vi "FieldMillTOBoltek.vi"() -> ()   [LabVIEW 2010]
uses:
  <vilib>/Utility/error.llb/DialogType.ctl
  <vilib>/Platform/TimedLoop/XDataNode/XDataNode.xnode
  <vilib>/Platform/TimedLoop/XDataNode/timing_clust.ctl
  <vilib>/Platform/TimedLoop/XDataNode/nitl_modes.ctl
  <vilib>/Platform/TimedLoop/XDataNode/wakeup.ctl
  <vilib>/Instr/_visa.llb/VISA Configure Serial Port (Instr).vi
  <vilib>/Utility/file.llb/Write To Spreadsheet File (DBL).vi
  <vilib>/Utility/file.llb/Read From Spreadsheet File (DBL).vi
  <vilib>/Platform/TimedLoop/XDataNode/XDNodeRunTimeDep.lvlib
panel:
  out "6":bool
  out "12":bool
  out "24":bool
  out "37":bool
  out "6_R":dbl(knob) caption="6" scale=0.0..10.0
  out "12_R":dbl(knob) caption="12" scale=0.0..10.0
  out "24_R":dbl(knob) caption="24" scale=0.0..10.0
  out "37_R":dbl(knob) caption="37" scale=0.0..10.0
  out "Strike distance Km":dbl
  in  "6 2":bool
  in  "12 2":bool
  in  "24 2":bool
  in  "37 2":bool
  out "kV/m tampone":dbl
  out "BOL IN":bool
  out "Offset":dbl format="%.1f"
  out "BOL OUT":bool
  out "SOCKET":bool
  out "FTP":bool
  out "Inver. sign":bool=TRUE
  out "Mediated v..":bool
  in  "FEM_ON_OFF":string
  out "Offset_p":i32 format="%.1f"
  out "Inverted_p":string
  out "Mediated_p":string
  out "User:":string
  out "Min":sgl caption="Min hour" format="%.3f"
  out "Max":sgl caption="Max hour" format="%.3f"
  out "Min":sgl caption="Min 10Min" format="%.3f"
  out "Max":sgl caption="Max 10Min" format="%.3f"
  out "Min":sgl caption="Min Midnight" format="%.3f"
  out "Max":sgl caption="Max Midnight" format="%.3f"
  out "Station Info graph":string
  out "Time & Date 2":timestamp format="%<%x>T"
  out "Time & Date":timestamp format="%<%H:%M:%S>T"
  out "String Alarm":string
  in  "About":bool
  in  "temp.csv midnight":bool
  out "remoteinfopath":string
  in  "Graph":bool=TRUE
  out "CLOSE COMMBOL":errorcluster
  out "CLOSE COMMFEM":errorcluster
  in  "COMMBOL ON_OFF":string
  out "Array via socket":string[](array[string])
  out "Multi socket String":string
  out "Alarm VHf counter":i32
  in  "Numero ripetizioni alarm VHf":i32
  out "In ripetizione VHf ?":bool
  out "Alarm Hf counter":i32
  in  "Numero ripetizioni alarm Hf":i32
  out "FEM Graph_IMAGES":cluster{dbl, dbl}[](graph) caption="FEM software - 5 min Graph - 15-05-13 / 11:59:33 ---- [ ROMA(Italy) - 41.995461 - 12.546161 - http://www.kwos.org ]"
  in  "SOCKET ON_OFF":string
  in  "Socket Port":u16=6340 min=1025 step=1
  out "Socket String":string
  out "24hour graph string":string
  out "4hour graph string":string
  out "1hour graph string":string
  out "LiveGraph string":string
  in  "Path24hourFile":path
  in  "Path4hourFile":path
  in  "Path1hourFile":path
  in  "PathCurrentFile":path
  in  "Ripetizioni alarm VHf":bool
  out "In allarme VHf ?":bool
  out "In allarme Hf ?":bool
  in  "Ripetizioni alarm Hf":bool
  out "Seconds Very High field alarm":sgl=1.0 format="%#_1f"
  out "Very High field alarm":sgl=5.0 format="%#_1f"
  out "Seconds High field alarm":sgl=1.0 format="%#_1f"
  out "High field alarm":sgl=1.0 format="%#_1f"
  in  "MENU ALARMS":bool
  out "Offset":dbl
  in  "Time Knob":u32(knob)=320 scale=300.0..86400.0 scale format="%#.0g"
  out "kV/m":string caption="kV/m display"
  out "FEM Graph":cluster{dbl, dbl}[](graph) caption="FEM software - 24 hours Graph - 23-10-09 / 18:44:02"
  in  "kV/m knob":sgl(knob)=1.0 scale=0.5..20.0
  out "data string 3":string
  out "data string FEM":string
  out "Mediated v.":bool
  out "Inversion sign":bool=TRUE caption="Inversion sign 2"
  out "FTP":bool
  in  "MENU INTERNET":bool
  in  "MENU FILTERS":bool
  out "Errori lettura file di configurazione":errorcluster={"status"=FALSE, "code"=0, "source"="Read File+ (string): Read File"}
  out "4 valori per media in array":dbl[](array[numeric]) format="%0.2f"
  in  "remotepath":string
  in  "passftp":string
  in  "loginftp":string
  in  "ftpsite":string
  in  "seconds":u32=30 min=30 max=3600 step=30
  in  "port number 2":refnum<visa-resource-name>="COM16"
  in  "parity 2":enum16{"None", "Odd", "Even", "Mark", "Space"}(ring)
  in  "port number":refnum<visa-resource-name>="COM5"
  in  "parity":enum16{"None", "Odd", "Even", "Mark", "Space"}(ring)
  out "COM err msg: 2":string="No Error"
  out "Boolean 2":bool
  in  "data bit 2":i32=8
  in  "baud rate 2":u32=9600
  out "kV/m":string
  out "mV":string
  in  "data bit":i32=8
  out "Boolean":bool
  in  "baud rate":u32=9600
  out "COM err msg:":string="No Error"
  # "E-Field Mill"
  # "kV/m"
  # "mV"
  # "=>"
  # "Sezione TEST"
  # "E-Field Mill Software"
  # "COMMFEM"
  # "COMMBOL"
  # "FILTRI"
  # "No"
  # "Yes"
  # "Inv"
  # "Norm"
  # "INTERNET"
  # "FTP TRANSFER ON/OFF"
  # "ALLARMI"
  # "Strike distance evaluation"
  # "Km"
  # "Last 10 min"
  # "Last hour"
  # "From midnight"
  # "ALERT Indicator"
  # "FEEDBACK RS232 => BOLTEK"
  # "FEEDBACK RS232 <= FEM"
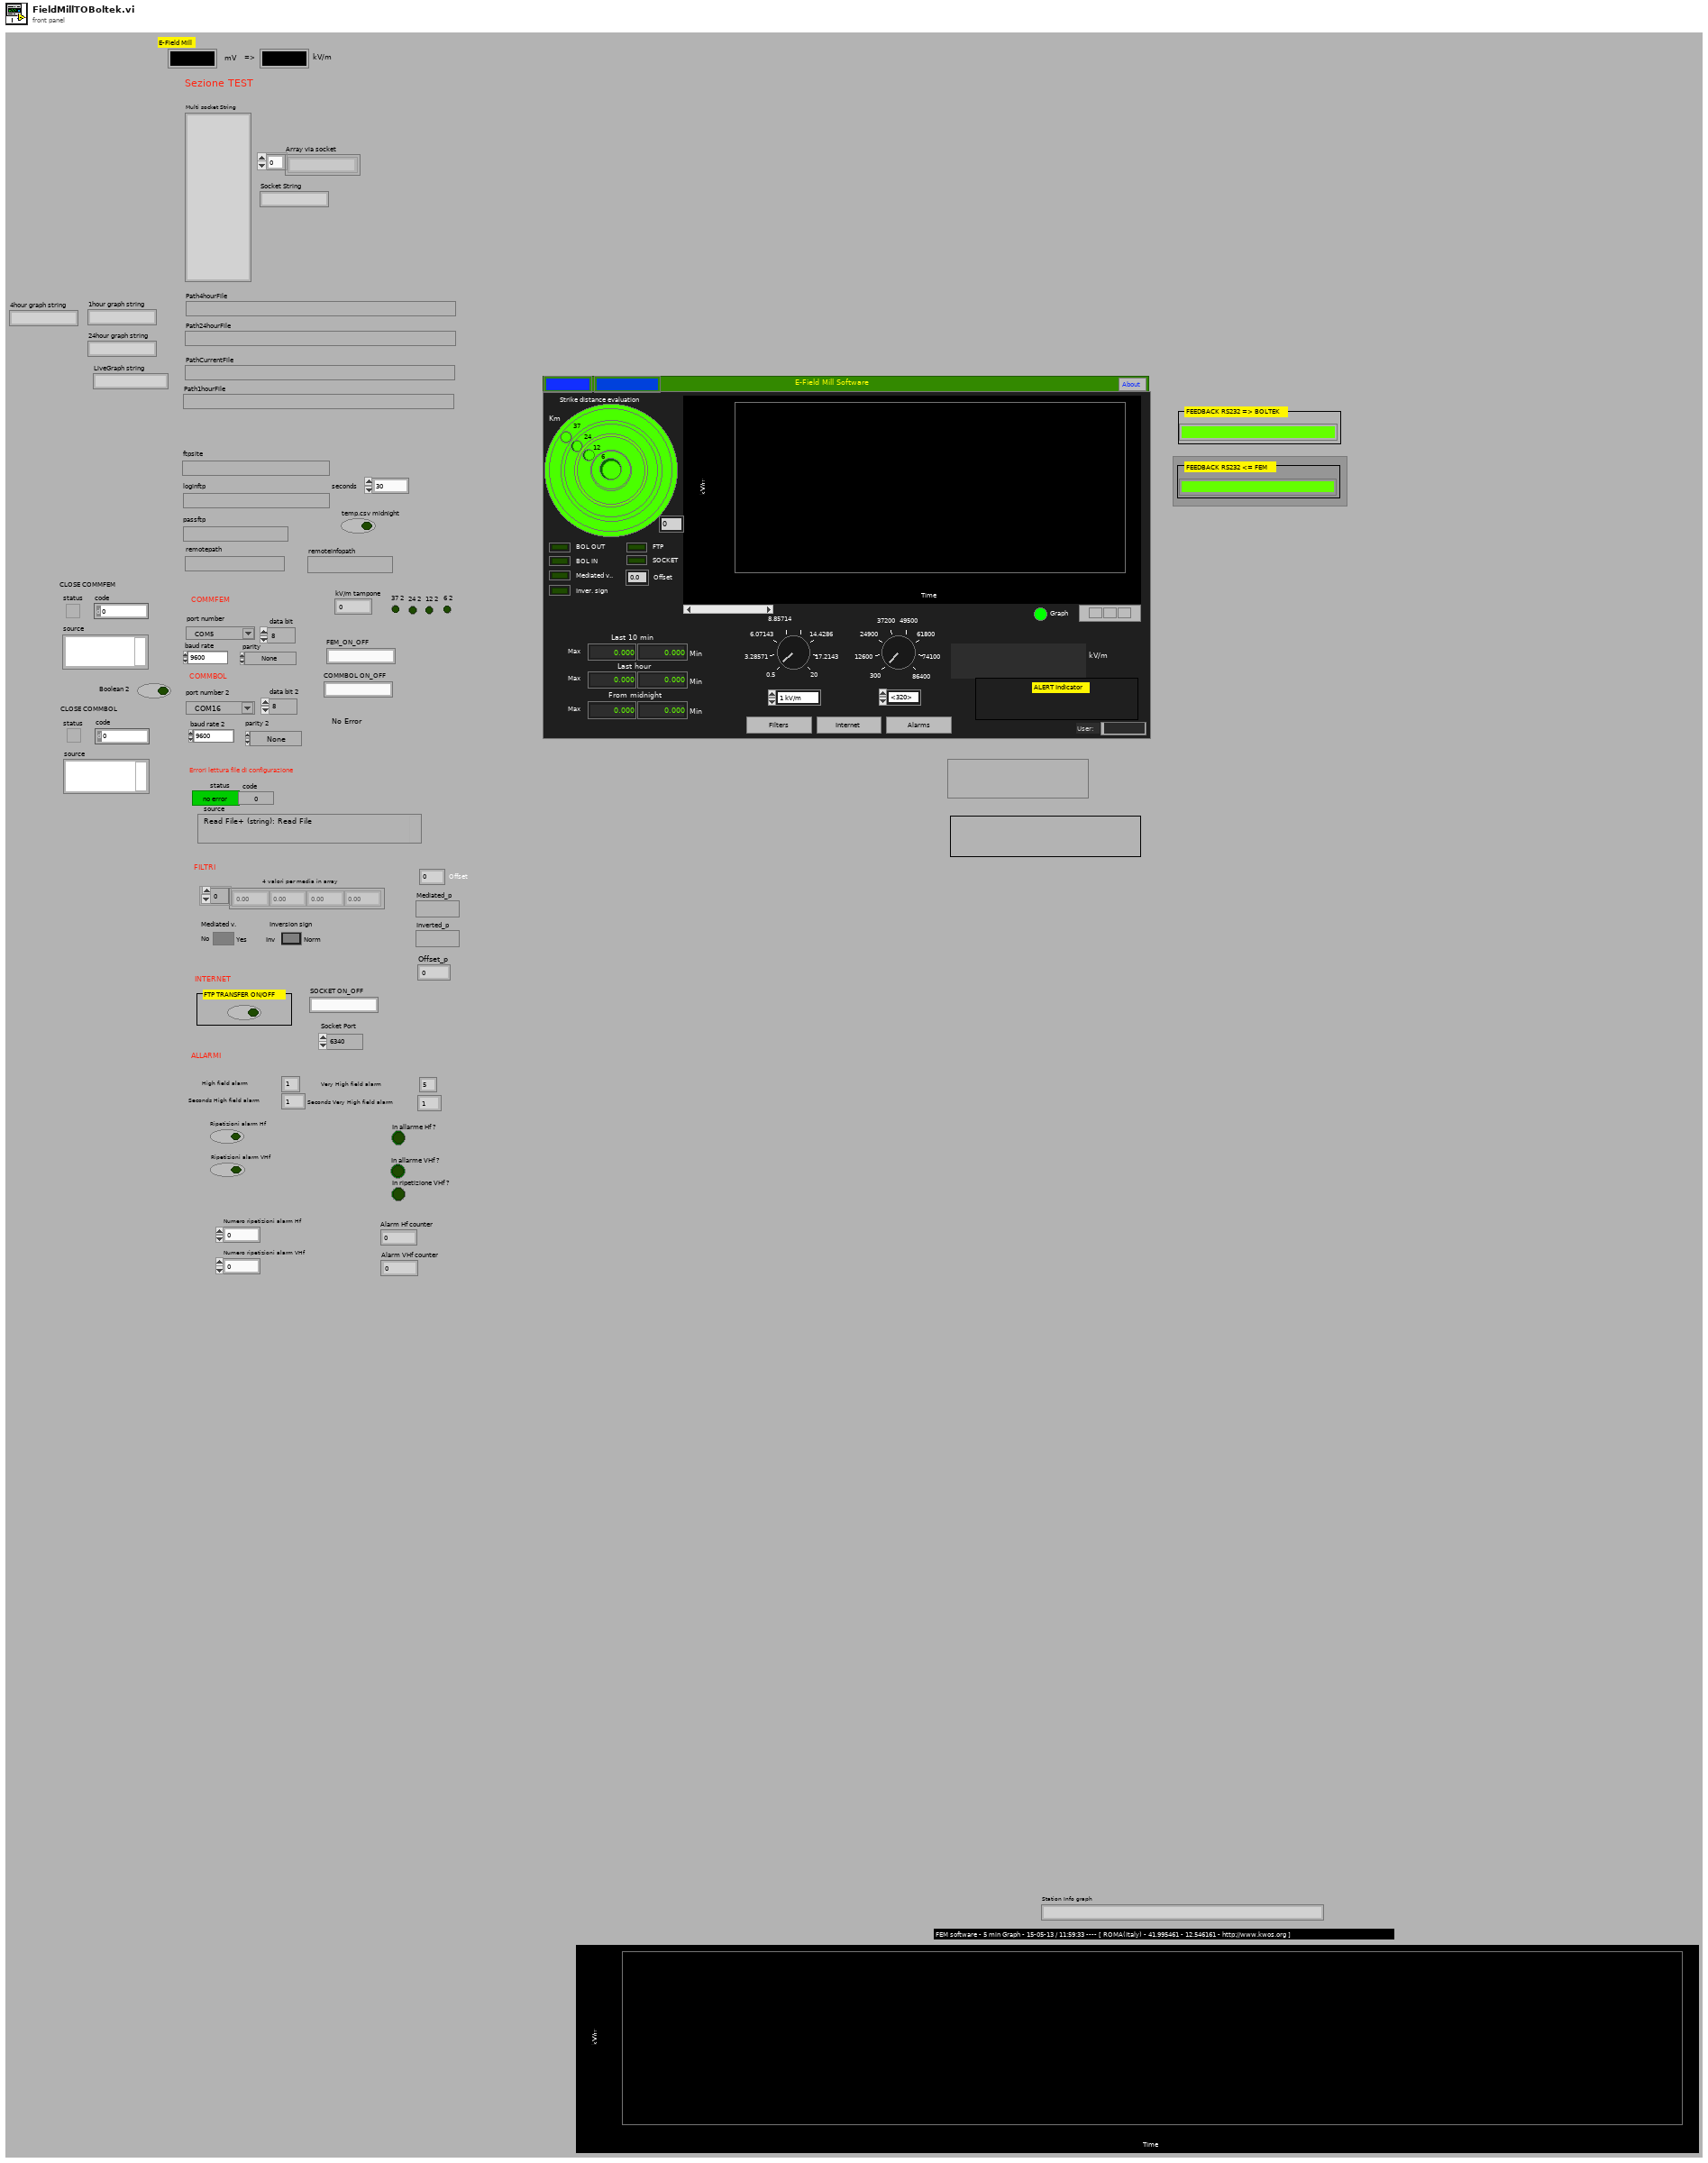
[diagram p1: front panel]
types:
  T1 = enum16{"open", "replace", "create", "open or create", "replace or create", "replace or create with confirmation"}
  T2 = typedef "XDNodeRunTimeDep.lvlib/timing_clust.ctl" = cluster{"Expected End [f-1]":u64, "Actual End [f-1]":u64, "Finished Late? [f-1]":bool, "Expected End [i-1]":u64, "Actual End [i-1]":u64, "Finished Late? [i-1]":bool, "Expected Start [i]":u64, "Actual Start [i]":u64, "Expected Start [f]":u64, "Actual Start [f]":u64, "Source Name":string, "Structure Name":string, "Period":i64, "Deadline":i64, "Offset":i64, "Start":i64, "Priority":i32, "Timeout":i32, "Mode":T3, "Wakeup Reason":T4, "Error":errorcluster, "Source Type":string, "Secondary Source Type":string, "Global End Time":u64, "Global Start Time":u64, "Frame Duration":u64, "Iteration Duration":u64, "Assigned CPU":i32, "I/O Scan Engine Mode":u32}
  T3 = typedef "XDNodeRunTimeDep.lvlib/nitl_modes.ctl" = enum32{"No Change", "Process missed periods, maintain original phase", "Discard missed periods, maintain original phase", "Process missed periods, ignore original phase", "Discard missed periods, ignore original phase"}
  T4 = typedef "XDNodeRunTimeDep.lvlib/wakeup.ctl" = enum32{"Normal", "Aborted", "Asynchronous wakeup", "Timing source error", "Timed loop error", "Timeout"}
  T5 = typedef "DialogType.ctl" = u16
  T6 = cluster{"second":i32, "minute":i32, "hour":i32, "day of month":i32, "month":i32, "year":i32, "day of week":i32, "day of year":i32, "is DST":i32}
  T7 = typedef "imagedata.ctl" = cluster{"image type":i32, "image depth":i32, "image":u8[], "mask":u8[], "colors":u32[], "Rectangle":cluster{"left":i16, "top":i16, "right":i16, "bottom":i16}}
  T8 = cluster{"Array via socket[0]":string, "Array via socket[1]":string, "Array via socket[2]":string, "Array via socket[3]":string, "Array via socket[4]":string, "Array via socket[5]":string, "Array via socket[6]":string, "Array via socket[7]":string, "Array via socket[8]":string, "Array via socket[9]":string, "Array via socket[10]":string, "Array via socket[11]":string, "Array via socket[12]":string, "Array via socket[13]":string, "Array via socket[14]":string}
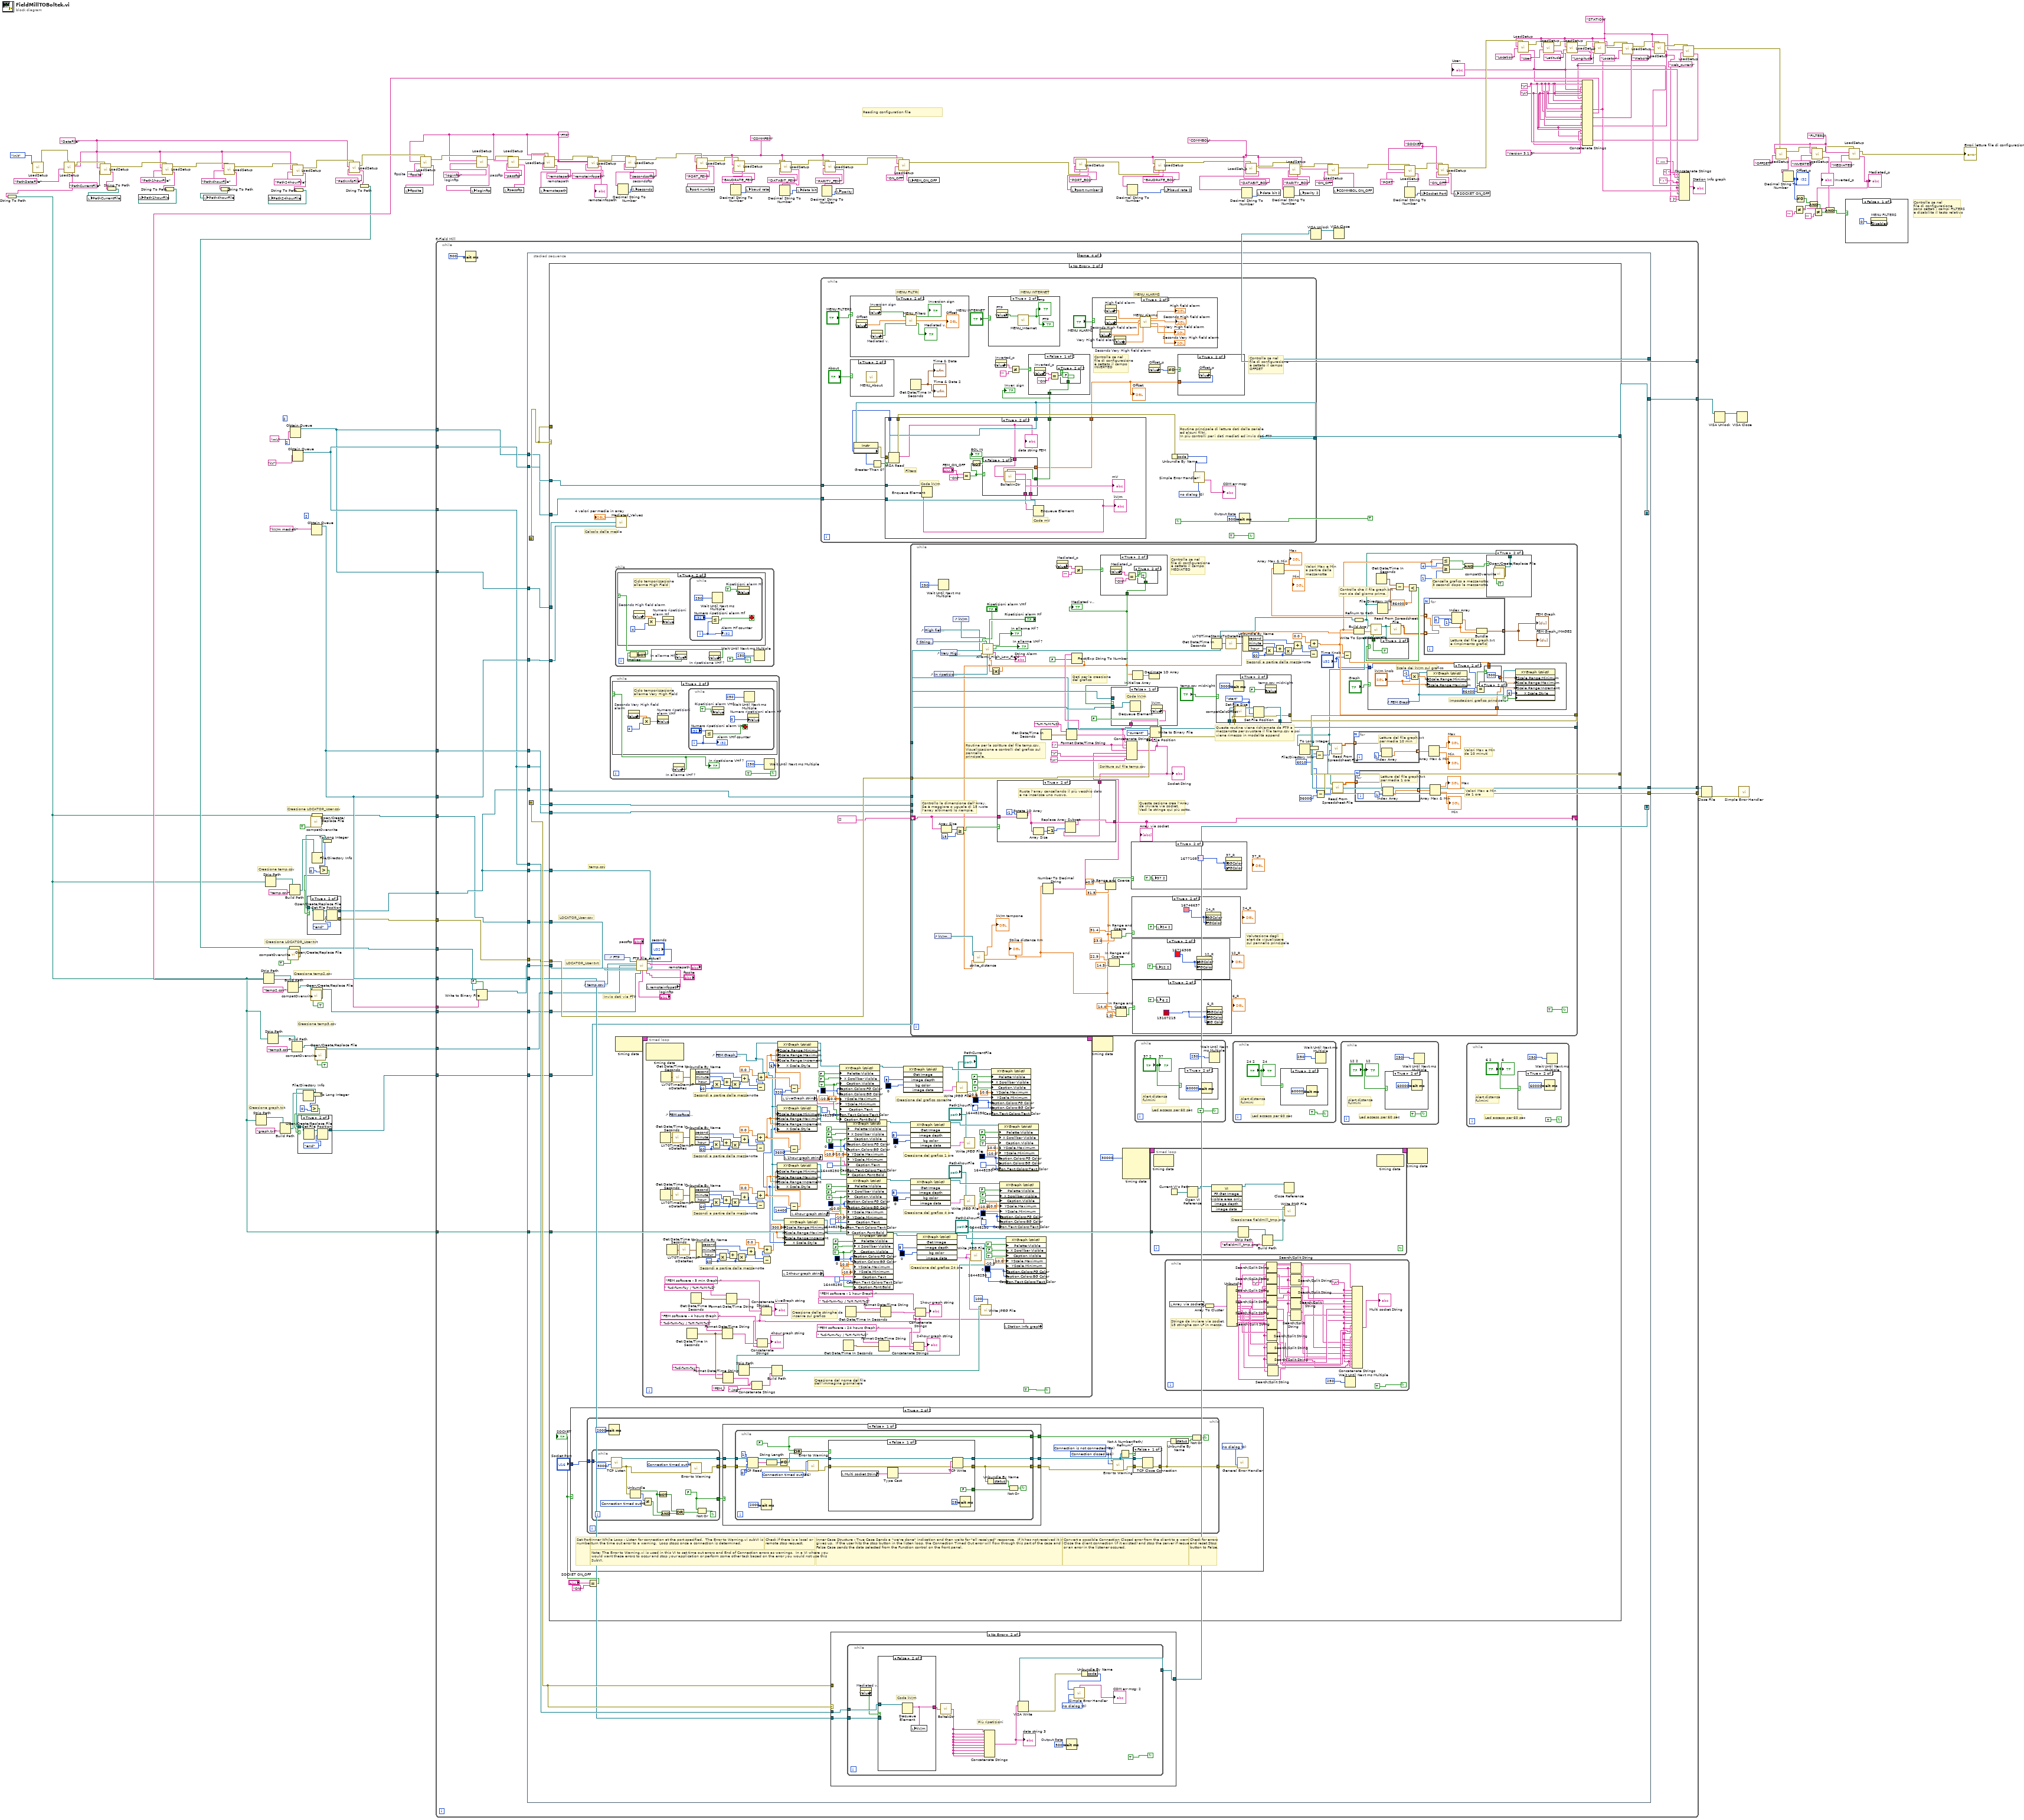
[diagram p0: block diagram]
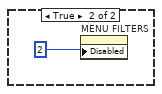
[diagram p2: hidden frame]
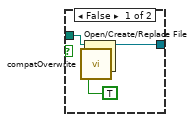
[diagram p3: hidden frame]
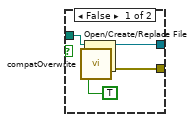
[diagram p4: hidden frame]
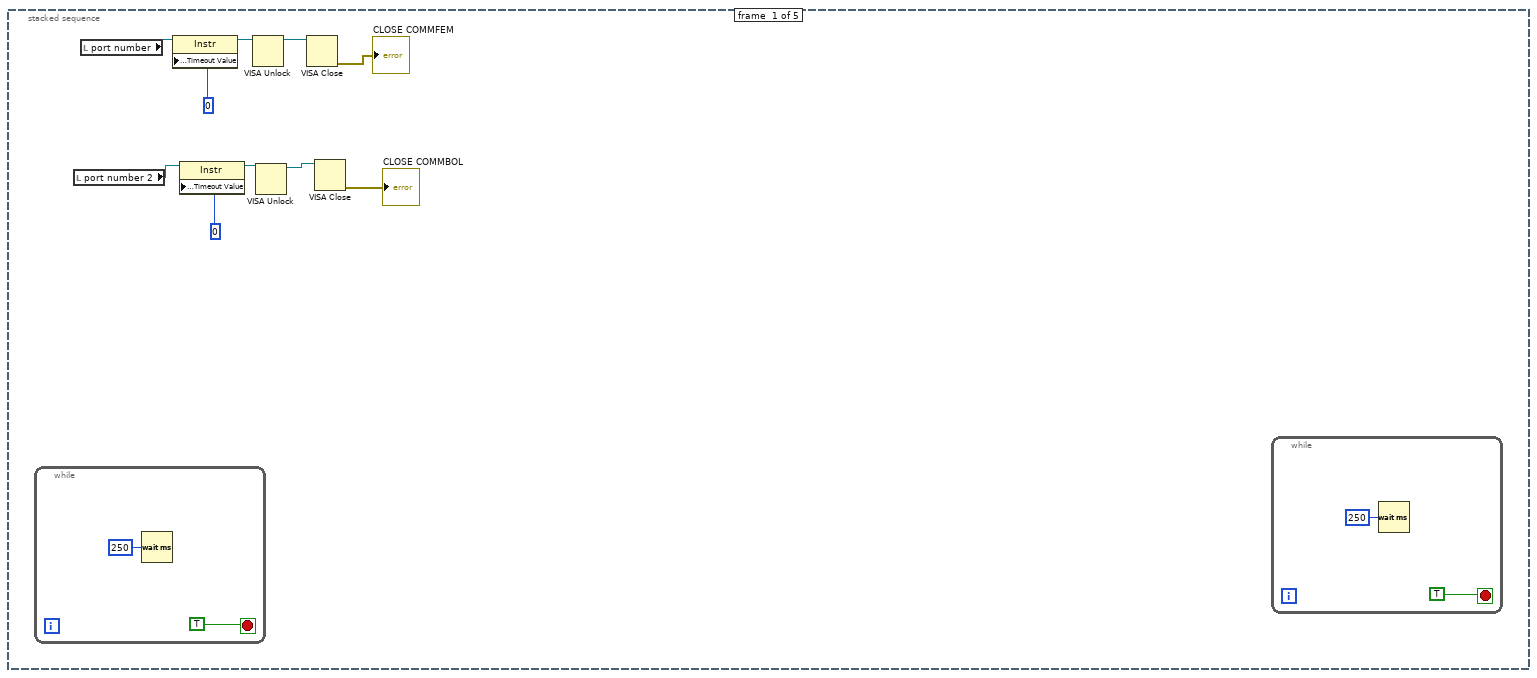
[diagram p5: hidden frame]
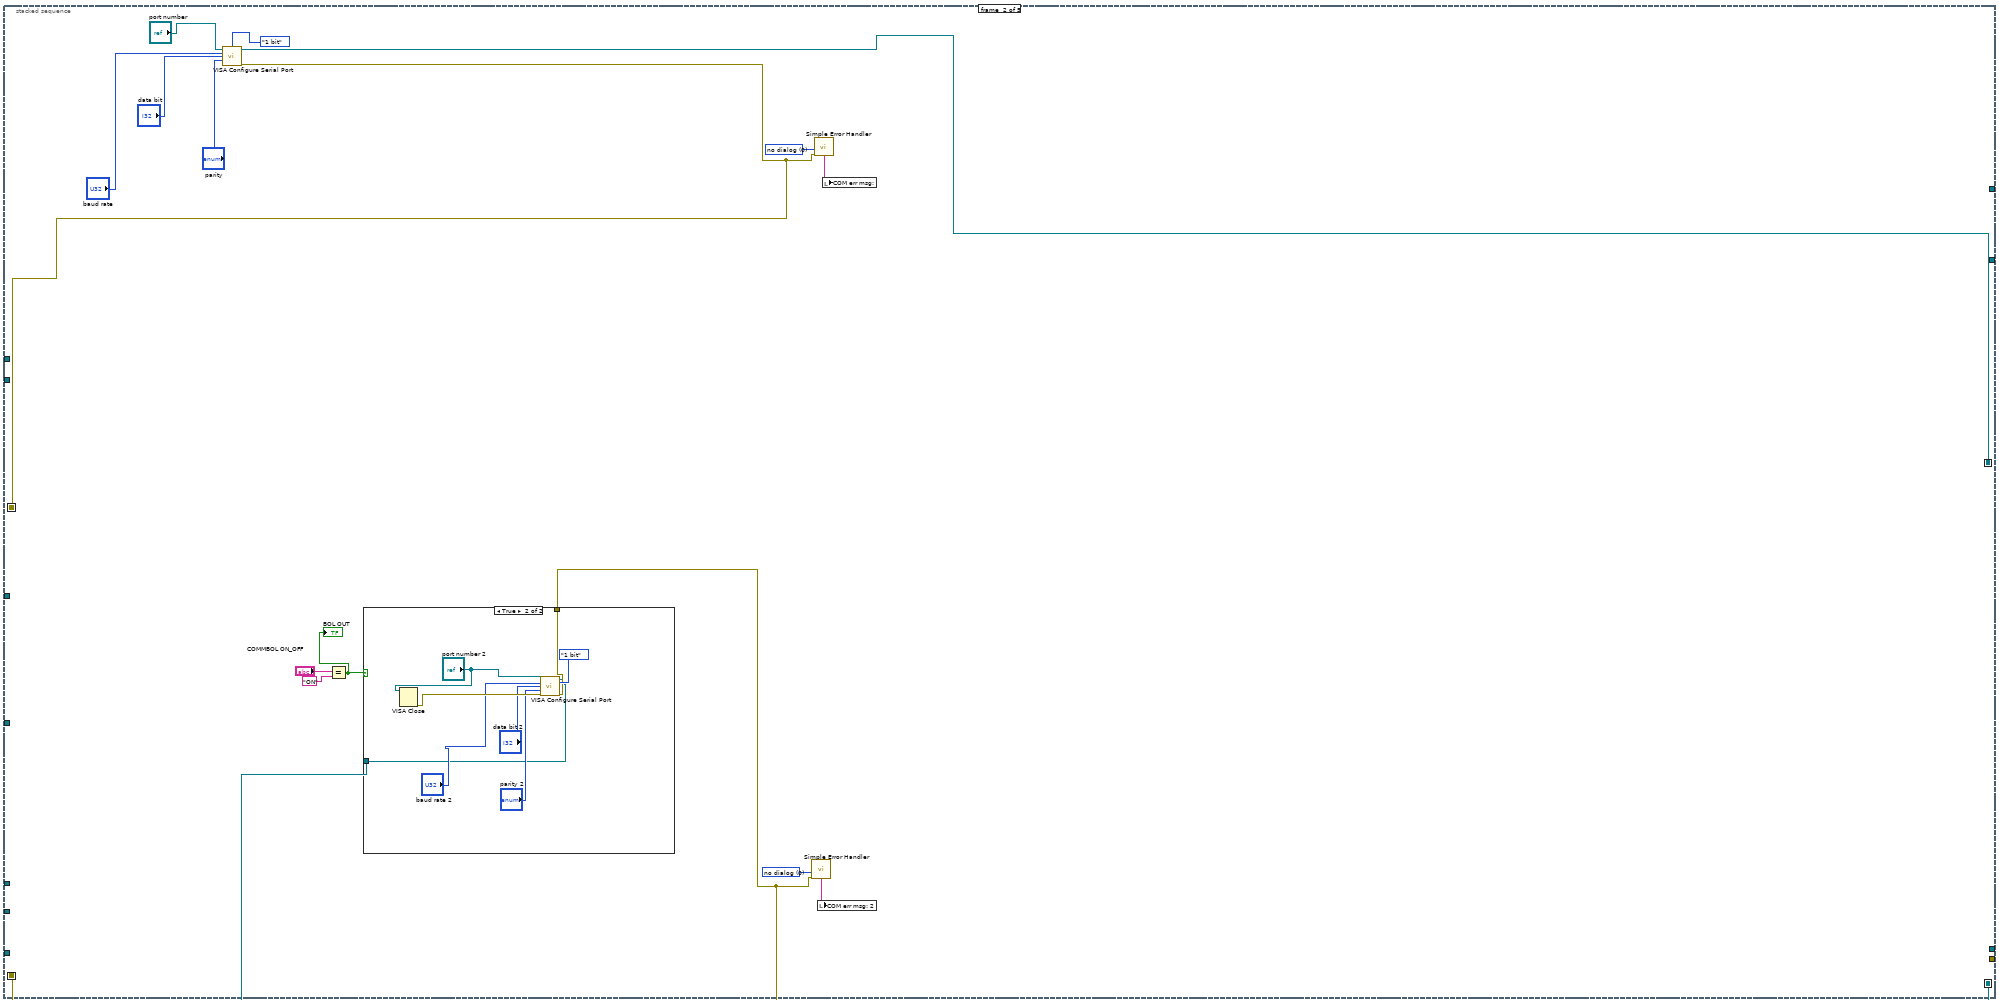
[diagram p6: hidden frame]
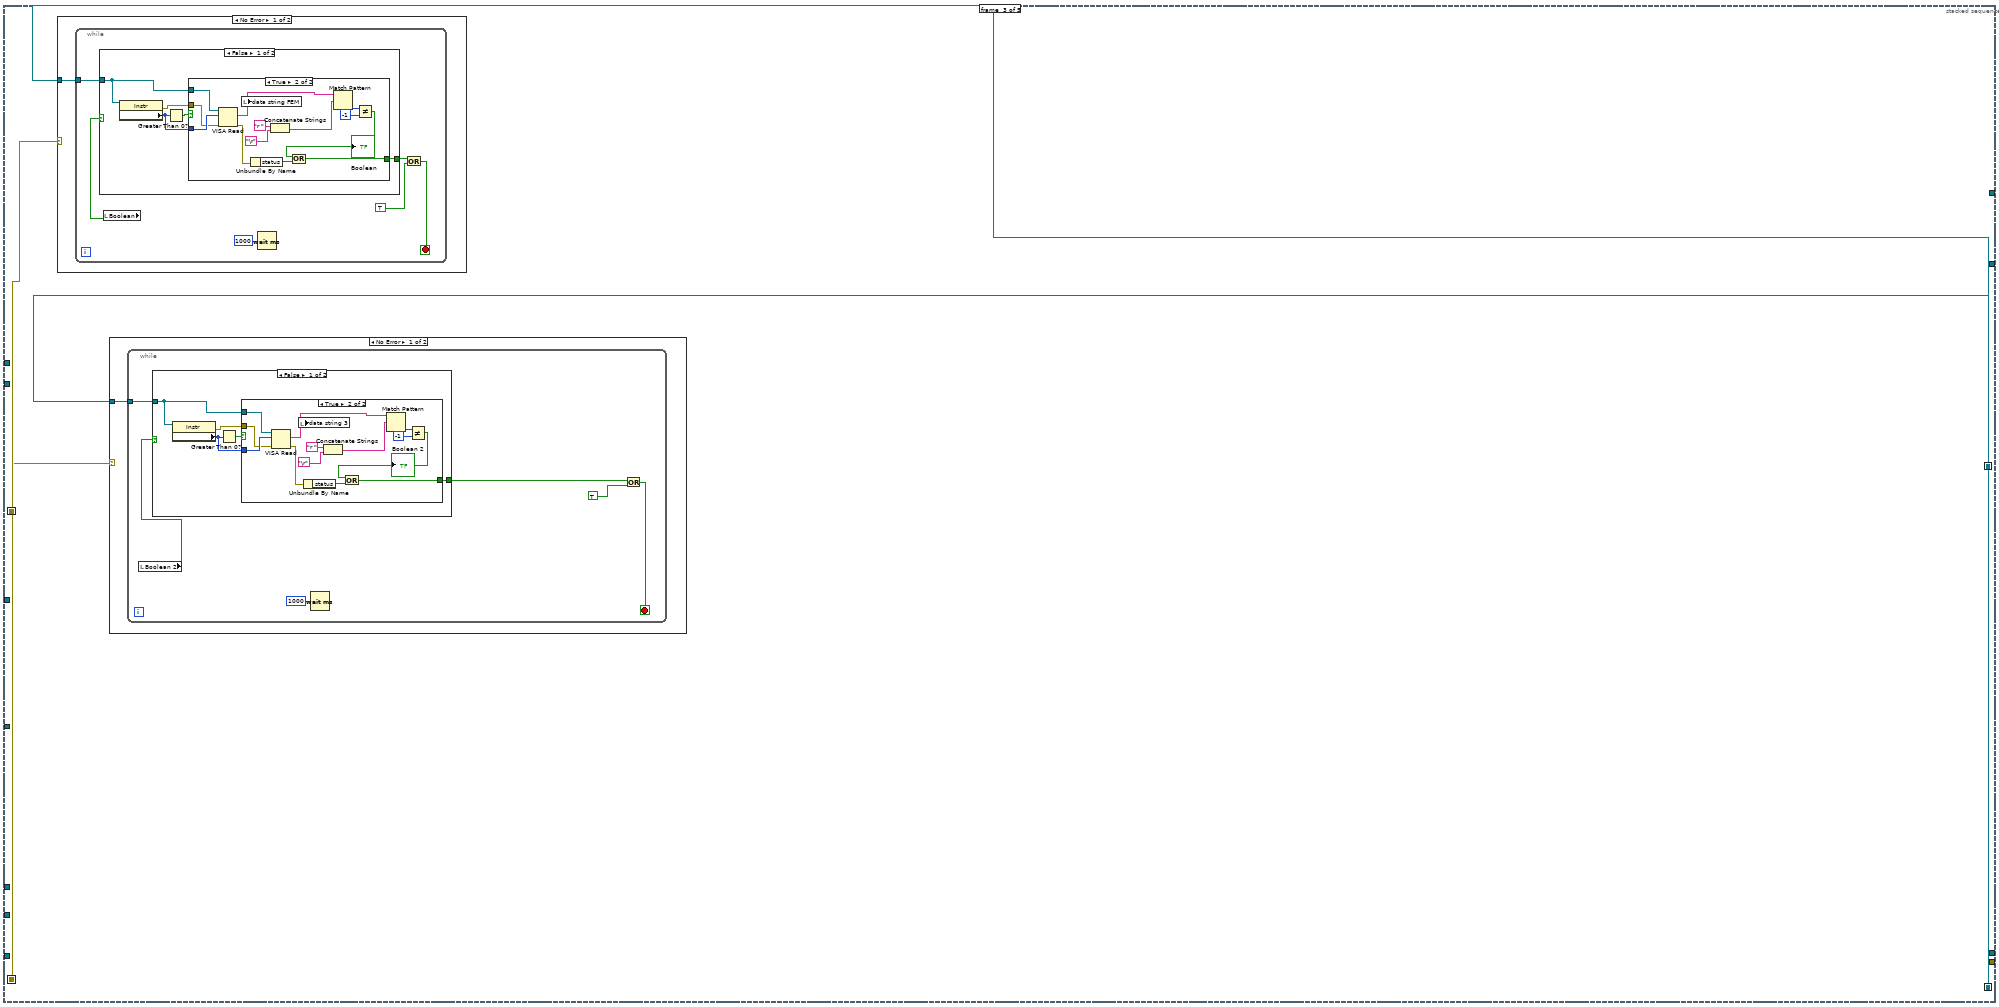
[diagram p8: hidden frame]
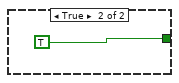
[diagram p10: hidden frame]
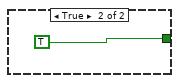
[diagram p13: hidden frame]
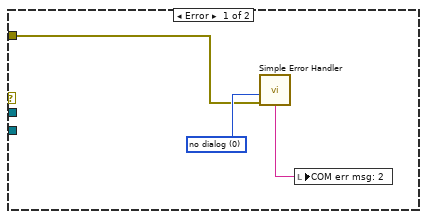
[diagram p15: hidden frame]
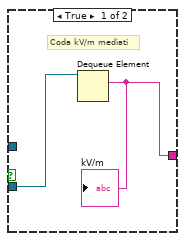
[diagram p16: hidden frame]
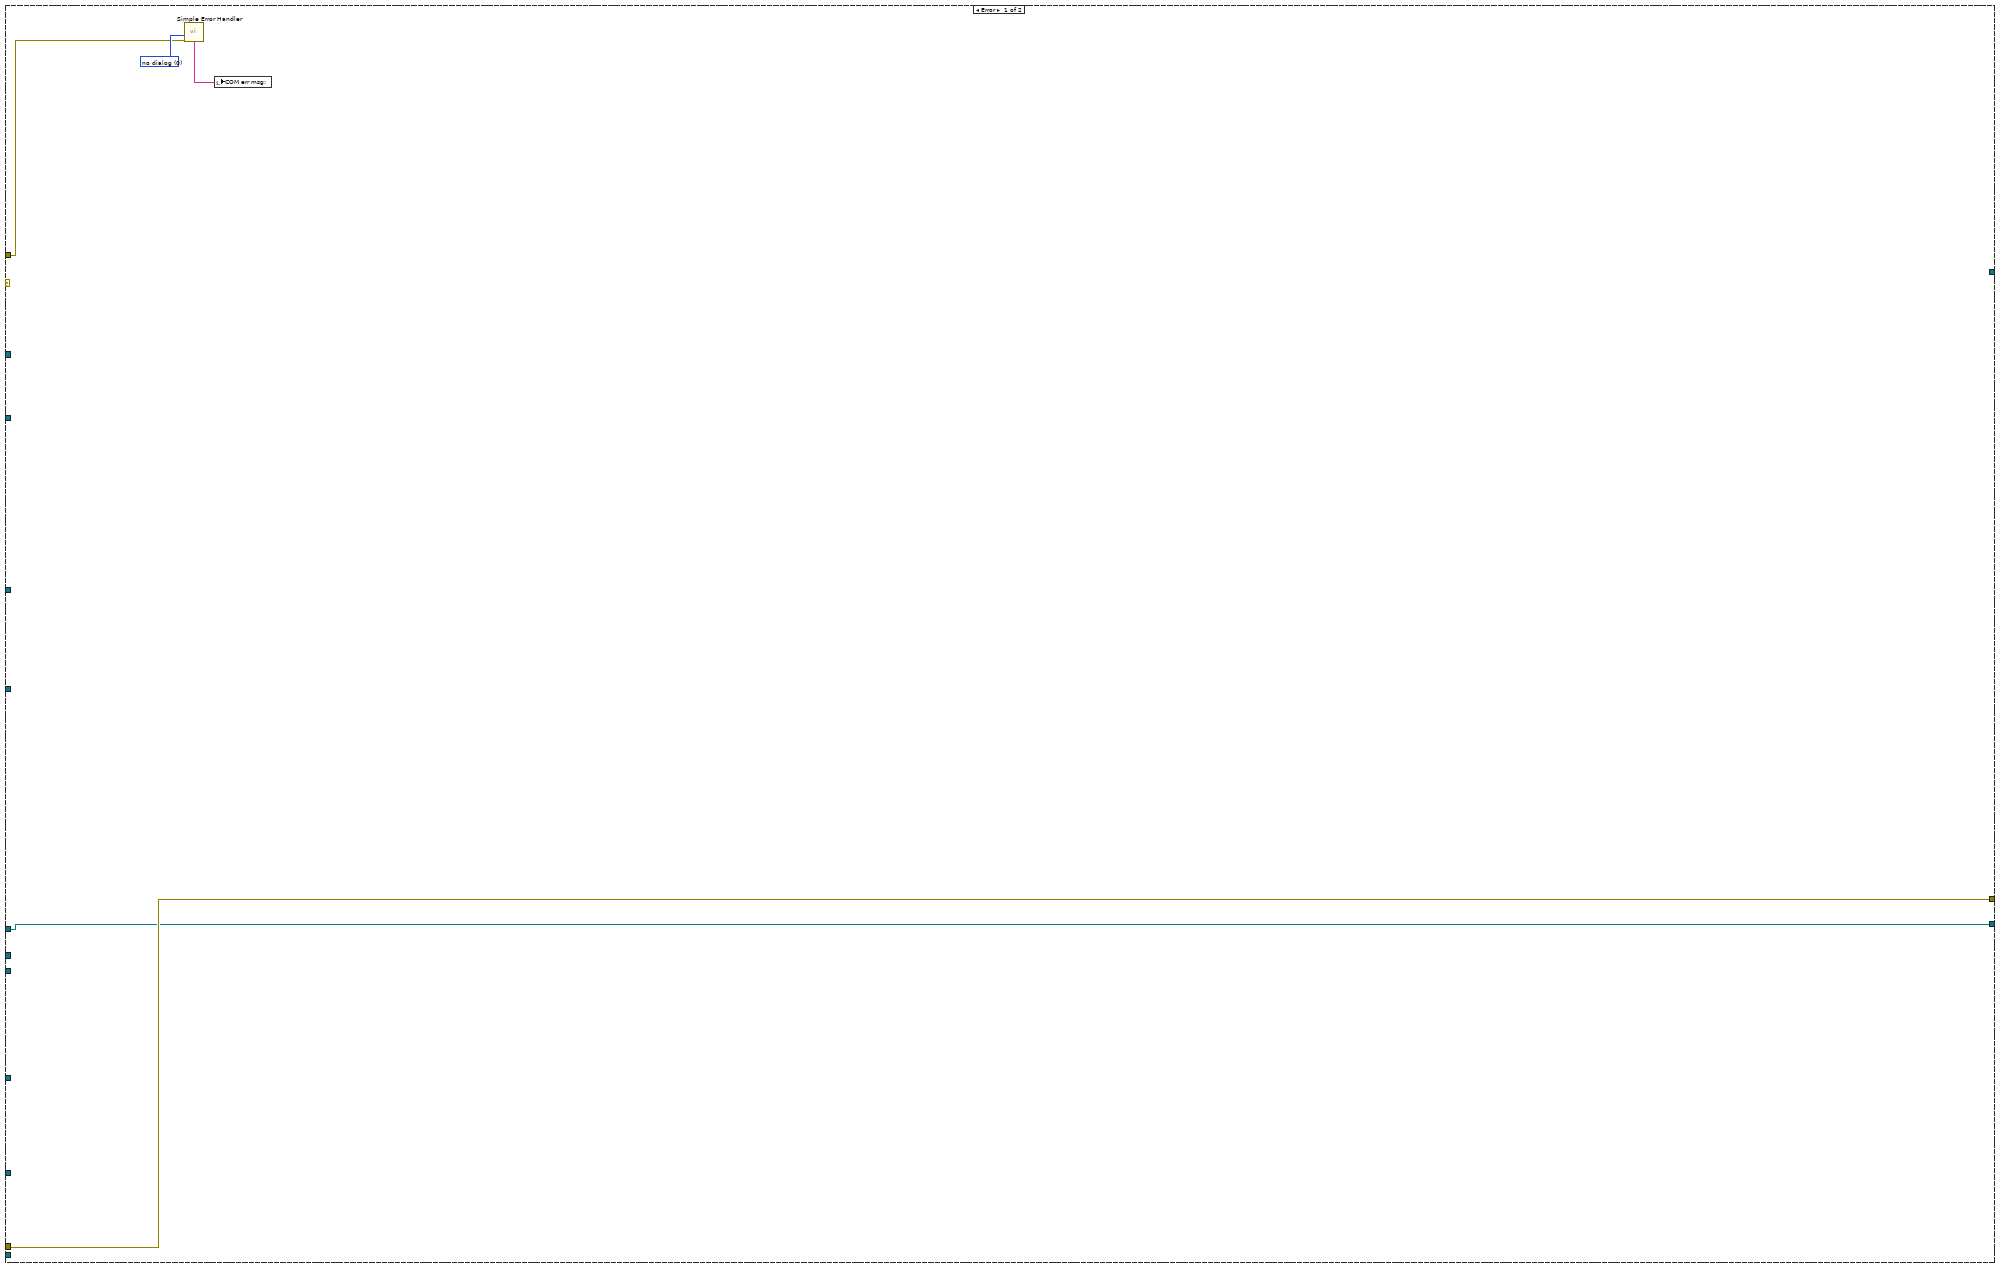
[diagram p17: hidden frame]
diagram:
  (unwired) 2 ("max queue size (-1, unlimited)")
  (unwired) 2 ("max queue size (-1, unlimited)")
  (unwired) 2 ("max queue size (-1, unlimited)")
  w32 = "FILTERS" ("section")
  w37 = " - " ("string")
  w49 = "\n"
  w50 = "\r"
  w48 = "STATION" ("section")
  w121 = "SOCKET" ("section")
  w112 = "COMMBOL" ("section")
  w3 = "COMMFEM" ("section")
  w174 = "secondsofftp"  # secondsftp
  w176 = "remotepath"  # remotepath
  w179 = "passftp"  # passftp
  w182 = "loginftp"  # loginftp
  w185 = "ftpsite"  # ftpsite
  w56 = "FTP" ("section")
  w88 = "DataFile" ("section")
  # "Controlla se nel\nfile di configurazione\nsono settati i campi FILTERS\ne disabilita il tasto relativo"
  # "Creazione temp3.csv"
  # "Creazione graph.txt"
  # "Creazione temp2.csv"
  # "Creazione LOCATOR_User.txt"
  # "Creazione temp.csv"
  # "Creazione LOCATOR_User.csv"
  # "Reading configuration file"
  n1 = call "LoadSetup.vi"("select"=enum16{"Init", "Read"}."Init") -> ("error out"=w186:errorcluster)  [unwired: 4 in, 1 out]
  n2 = call "LoadSetup.vi"("section"=w88, "key"="PathDataFile" ("PathDataFile"), "error in (not an error)"=w186) -> ("error out"=w137:errorcluster, "value"=w170:string)  [unwired: 2 in]
  n3 = String To Path(string=w170) -> (path=w1:path)
  n4 = call "LoadSetup.vi"("section"=w88, "key"="PathCurrentFile" ("PathCurrentFile"), "error in (not an error)"=w137) -> ("error out"=w134:errorcluster, "value"=w138:string)  [unwired: 2 in]
  n5 = String To Path(string=w138) -> (path=w135:path)
  n6 = local write "PathCurrentFile"(w135) -> ()
  n7 = call "LoadSetup.vi"("section"=w88, "key"="Path1hourFile" ("Path1hourFile"), "error in (not an error)"=w134) -> ("error out"=w128:errorcluster, "value"=w133:string)  [unwired: 2 in]
  n8 = String To Path(string=w133) -> (path=w131:path)
  n9 = local write "Path1hourFile"(w131) -> ()
  n10 = call "LoadSetup.vi"("section"=w88, "key"="Path4hourFile" ("Path1hourFile"), "error in (not an error)"=w128) -> ("error out"=w125:errorcluster, "value"=w129:string)  [unwired: 2 in]
  n11 = String To Path(string=w129) -> (path=w127:path)
  n12 = local write "Path4hourFile"(w127) -> ()
  n13 = Strip Path(path=w1) -> (stripped path=w64:path)  [unwired: 1 out]
  n14 = Strip Path(path=w1) -> (stripped path=w73:path)  [unwired: 1 out]
  n15 = Strip Path(path=w1) -> (stripped path=w83:path)  [unwired: 1 out]
  n16 = Strip Path(path=w1) -> (stripped path=w46:path)  [unwired: 1 out]
  n17 = Build Path(base path=w64, name or relative path="graph.txt") -> (appended path=w60:path)
  n18 = Build Path(base path=w73, name or relative path="temp2.csv") -> (appended path=w74:path)
  n19 = call <vilib>:"compatOverwrite.vi"("overwrite (F)"=TRUE) -> ("overwrite?"=w9:T1)
  n20 = Build Path(base path=w83, name or relative path="temp.csv") -> (appended path=w67:path)
  n21 = Obtain Queue(element data type="mV") -> (queue out=w139:refnum<queue>)  [unwired: 4 in, 2 out]
  n22 = Build Path(base path=w46, name or relative path="temp3.csv") -> (appended path=w47:path)
  n23 = Obtain Queue(element data type="kV") -> (queue out=w191:refnum<queue>)  [unwired: 4 in, 2 out]
  n24 = call "LoadSetup.vi"("section"=w88, "key"="Path24hourFile" ("Path1hourFile"), "error in (not an error)"=w125) -> ("error out"=w90:errorcluster, "value"=w124:string)  [unwired: 2 in]
  n25 = String To Path(string=w124) -> (path=w123:path)
  n26 = local write "Path24hourFile"(w123) -> ()
  n27 = File/Directory Info(path=w60) -> (path out=w59:path, size=w12:i64)  [unwired: 1 in, 5 out]
  n28 = call <vilib>:"compatOverwrite.vi"("overwrite (F)"=TRUE) -> ("overwrite?"=w8:T1)
  n29 = call <vilib>:"compatOverwrite.vi"("overwrite (F)"=TRUE) -> ("overwrite?"=w10:T1)
  n30 = Obtain Queue(element data type="kV/m mediati") -> (queue out=w140:refnum<queue>)  [unwired: 4 in, 2 out]
  n31 = Open/Create/Replace File(file path (use dialog)=w1, operation (0:open)=w8) -> (refnum out=w78:refnum<file>)  [unwired: 4 in, 2 out]
  n32 = Open/Create/Replace File(file path (use dialog)=w74, operation (0:open)=w10) -> (refnum out=w70:refnum<file>)  [unwired: 4 in, 2 out]
  n33 = File/Directory Info(path=w67) -> (path out=w66:path, size=w11:i64)  [unwired: 1 in, 5 out]
  n34 = To Long Integer(number=w12) -> (32bit integer=w61:i32)
  n35 = Greater?(x=w61, y=0) -> (0:w58:bool)
  n36 = case shown="True" w58 {
    tunnel: w59 -> [w196 w200]
    tunnel: [w194 w198] -> w57
    frame False {
      n37 = call <vilib>:"compatOverwrite.vi"("overwrite (F)"=TRUE) -> ("overwrite?"=w193:T1)
      n38 = Open/Create/Replace File(file path (use dialog)=w196, operation (0:open)=w193) -> (refnum out=w194:refnum<file>)  [unwired: 4 in, 2 out]
    }
    frame True {
      n39 = Open/Create/Replace File(file path (use dialog)=w200) -> (refnum out=w199:refnum<file>)  [unwired: 5 in, 2 out]
      n40 = Set File Position(refnum=w199, from (0:start)=enum16{"start", "end", "current"}."end" ("pos mode (0:1)")) -> (refnum out=w198:refnum<file>)  [unwired: 2 in, 1 out]
    }
  }
  n41 = call <vilib>:"compatOverwrite.vi"("overwrite (F)"=TRUE) -> ("overwrite?"=w13:T1)
  n42 = Open/Create/Replace File(file path (use dialog)=w47, operation (0:open)=w13) -> (refnum out=w43:refnum<file>)  [unwired: 4 in, 2 out]
  n43 = To Long Integer(number=w11) -> (32bit integer=w68:i32)
  n44 = Greater?(x=w68, y=0) -> (0:w65:bool)
  n45 = case shown="True" w65 {
    tunnel: w66 -> [w205 w211]
    tunnel: [w203 w209] -> w81
    tunnel: [w202 w207] -> w80
    frame False {
      n46 = call <vilib>:"compatOverwrite.vi"("overwrite (F)"=TRUE) -> ("overwrite?"=w201:T1)
      n47 = Open/Create/Replace File(file path (use dialog)=w205, operation (0:open)=w201) -> (refnum out=w203:refnum<file>, error out=w202:errorcluster)  [unwired: 4 in, 1 out]
    }
    frame True {
      n48 = Open/Create/Replace File(file path (use dialog)=w211) -> (refnum out=w210:refnum<file>, error out=w208:errorcluster)  [unwired: 5 in, 1 out]
      n49 = Set File Position(refnum=w210, from (0:start)=enum16{"start", "end", "current"}."end" ("pos mode (0:1)"), error in=w208) -> (refnum out=w209:refnum<file>, error out=w207:errorcluster)  [unwired: 1 in]
    }
  }
  n50 = call "LoadSetup.vi"("section"=w88, "key"="PathInfoFile" ("PathDataFile"), "error in (not an error)"=w90) -> ("error out"=w89:errorcluster, "value"=w86:string)  [unwired: 2 in]
  n51 = String To Path(string=w86) -> (path=w75:path)
  n52 = Open/Create/Replace File(file path (use dialog)=w75, operation (0:open)=w9) -> (refnum out=w76:refnum<file>)  [unwired: 4 in, 2 out]
  n53 = call "LoadSetup.vi"("section"=w56, "key"=w185, "error in (not an error)"=w89) -> ("error out"=w183:errorcluster, "value"=w184:string)  [unwired: 2 in]
  n54 = local write "ftpsite"(w184) -> ()
  n55 = call "LoadSetup.vi"("section"=w56, "key"=w182, "error in (not an error)"=w183) -> ("error out"=w180:errorcluster, "value"=w181:string)  [unwired: 2 in]
  n56 = local write "loginftp"(w181) -> ()
  n57 = call "LoadSetup.vi"("section"=w56, "key"=w179, "error in (not an error)"=w180) -> ("error out"=w177:errorcluster, "value"=w178:string)  [unwired: 2 in]
  n58 = local write "passftp"(w178) -> ()
  n59 = call "LoadSetup.vi"("section"=w56, "key"=w176, "error in (not an error)"=w177) -> ("error out"=w93:errorcluster, "value"=w175:string)  [unwired: 2 in]
  n60 = local write "remotepath"(w175) -> ()
  n61 = call "LoadSetup.vi"("section"=w56, "key"="remoteinfopath", "error in (not an error)"=w93) -> ("error out"=w92:errorcluster, "value"=→"remoteinfopath":string)  [unwired: 2 in]
  n62 = call "LoadSetup.vi"("section"=w56, "key"=w174, "error in (not an error)"=w92) -> ("error out"=w55:errorcluster, "value"=w172:string)  [unwired: 2 in]
  n63 = Decimal String To Number(string=w172) -> (number=w173:i32)  [unwired: 2 in, 1 out]
  n64 = local write "seconds"(w173) -> ()
  n65 = call "LoadSetup.vi"("section"=w3, "key"="PORT_FEM", "error in (not an error)"=w55) -> ("error out"=w167:errorcluster, "value"=w168:string)  [unwired: 2 in]
  n66 = local write "port number"(w168) -> ()
  n67 = call "LoadSetup.vi"("section"=w3, "key"="BAUDRATE_FEM", "error in (not an error)"=w167) -> ("error out"=w163:errorcluster, "value"=w165:string)  [unwired: 2 in]
  n68 = Decimal String To Number(string=w165) -> (number=w164:i32)  [unwired: 2 in, 1 out]
  n69 = local write "baud rate"(w164) -> ()
  n70 = call "LoadSetup.vi"("section"=w3, "key"="DATABIT_FEM", "error in (not an error)"=w163) -> ("error out"=w159:errorcluster, "value"=w160:string)  [unwired: 2 in]
  n71 = Decimal String To Number(string=w160) -> (number=w161:i32)  [unwired: 2 in, 1 out]
  n72 = local write "data bit"(w161) -> ()
  n73 = call "LoadSetup.vi"("section"=w3, "key"="PARITY_FEM", "error in (not an error)"=w159) -> ("error out"=w6:errorcluster, "value"=w156:string)  [unwired: 2 in]
  n74 = Decimal String To Number(string=w156) -> (number=w157:i32)  [unwired: 2 in, 1 out]
  n75 = local write "parity"(w157) -> ()
  n76 = call "LoadSetup.vi"("section"=w3, "key"="ON_OFF", "error in (not an error)"=w6) -> ("error out"=w5:errorcluster, "value"=w2:string)  [unwired: 2 in]
  n77 = local write "FEM_ON_OFF"(w2) -> ()
  n78 = call "LoadSetup.vi"("section"=w112, "key"="PORT_BOL", "error in (not an error)"=w5) -> ("error out"=w152:errorcluster, "value"=w154:string)  [unwired: 2 in]
  n79 = local write "port number 2"(w154) -> ()
  n80 = call "LoadSetup.vi"("section"=w112, "key"="BAUDRATE_BOL", "error in (not an error)"=w152) -> ("error out"=w7:errorcluster, "value"=w150:string)  [unwired: 2 in]
  n81 = Decimal String To Number(string=w150) -> (number=w151:i32)  [unwired: 2 in, 1 out]
  n82 = local write "baud rate 2"(w151) -> ()
  n83 = call "LoadSetup.vi"("section"=w112, "key"="DATABIT_BOL", "error in (not an error)"=w7) -> ("error out"=w143:errorcluster, "value"=w147:string)  [unwired: 2 in]
  n84 = Decimal String To Number(string=w147) -> (number=w148:i32)  [unwired: 2 in, 1 out]
  n85 = local write "data bit 2"(w148) -> ()
  n86 = call "LoadSetup.vi"("section"=w112, "key"="PARITY_BOL", "error in (not an error)"=w143) -> ("error out"=w115:errorcluster, "value"=w145:string)  [unwired: 2 in]
  n87 = Decimal String To Number(string=w145) -> (number=w144:i32)  [unwired: 2 in, 1 out]
  n88 = local write "parity 2"(w144) -> ()
  n89 = call "LoadSetup.vi"("section"=w112, "key"="ON_OFF", "error in (not an error)"=w115) -> ("error out"=w114:errorcluster, "value"=w111:string)  [unwired: 2 in]
  n90 = local write "COMMBOL ON_OFF"(w111) -> ()
  n91 = call "LoadSetup.vi"("section"=w121, "key"="PORT", "error in (not an error)"=w114) -> ("error out"=w122:errorcluster, "value"=w118:string)  [unwired: 2 in]
  n92 = Decimal String To Number(string=w118) -> (number=w117:i32)  [unwired: 2 in, 1 out]
  n93 = local write "Socket Port"(w117) -> ()
  n94 = call "LoadSetup.vi"("section"=w121, "key"="ON_OFF", "error in (not an error)"=w122) -> ("error out"=w100:errorcluster, "value"=w116:string)  [unwired: 2 in]
  n95 = local write "SOCKET ON_OFF"(w116) -> ()
  n96 = call "LoadSetup.vi"("section"=w48, "key"="Location", "error in (not an error)"=w100) -> ("error out"=w99:errorcluster, "value"=w40:string)  [unwired: 2 in]
  n97 = call "LoadSetup.vi"("section"=w48, "key"="User", "error in (not an error)"=w99) -> ("error out"=w98:errorcluster, "value"=w42:string)  [unwired: 2 in]
  "User:" <- w42
  n98 = call "LoadSetup.vi"("section"=w48, "key"="Latitude", "error in (not an error)"=w98) -> ("error out"=w97:errorcluster, "value"=w39:string)  [unwired: 2 in]
  n99 = call "LoadSetup.vi"("section"=w48, "key"="Longitude", "error in (not an error)"=w97) -> ("error out"=w96:errorcluster, "value"=w38:string)  [unwired: 2 in]
  n100 = call "LoadSetup.vi"("section"=w48, "key"="Locator", "error in (not an error)"=w96) -> ("error out"=w95:errorcluster, "value"=w94:string)  [unwired: 2 in]
  n101 = call "LoadSetup.vi"("section"=w48, "key"="Website", "error in (not an error)"=w95) -> ("error out"=w53:errorcluster, "value"=w36:string)  [unwired: 2 in]
  n102 = Concatenate Strings(" ---- " ("string"), "[ " ("string"), w40, w37, w39, w37, w38, w37, w36, " ]" ("string")) -> (→"Station Info graph":string)
  n103 = call "LoadSetup.vi"("section"=w48, "key"="web_current", "error in (not an error)"=w53) -> ("error out"=w26:errorcluster, "value"=w52:string)  [unwired: 2 in]
  n104 = Concatenate Strings(w40, w50, w49, w42, w50, w49, w39, w50, w49, w38, w50, w49, w94, w50, w49, w36, w50, w49, w52, w50, w49, "Version 3.1.3", w50, w49) -> (w84:string)
  n105 = while "E-Field Mill" {
    tunnel: [w234] -> w107
    tunnel: [w233] -> w109
    tunnel: w191 -> [w224]
    tunnel: w191 -> [w232]
    tunnel: w139 -> [w231]
    tunnel: w139 -> [w230]
    tunnel: w140 -> [w229]
    tunnel: w140 -> [w228]
    tunnel: [w227] -> w142
    tunnel: [w226] -> w141
    tunnel: w140 -> [w225]
    tunnel: w84 -> [w221]
    tunnel: w81 -> [w220]
    tunnel: w80 -> [w219]
    tunnel: w78 -> [w218]
    tunnel: w76 -> [w217]
    tunnel: w70 -> [w216]
    tunnel: w57 -> [w215]
    tunnel: w43 -> [w214]
    tunnel: w1 -> [w212]
    stop <- TRUE continue-if-true
    n106 = Wait (ms)(milliseconds to wait=500) -> ()  [unwired: 1 out]
    n107 = Write to Binary File ("Write File")(file (use dialog)=w217, data=w221, 5:FALSE ("prepend array or string size? (T)")) -> (refnum out=w222:refnum<file>)  [unwired: 3 in, 2 out]
    n108 = stacked-sequence {
      seq-local: [_ w259 _ _ _] -> [_ _ w277 w350 _]
      seq-local: [_ w262 _ _ _] -> [_ _ w276 w354 w1055]
      seq-local: [_ w254 _ _ _] -> [_ _ w275 w353 w1054]
      seq-local: [_ w255 _ _ _] -> [_ _ w274 w349 _]
      tunnel: [_ _ _ _ w1055] -> w234
      tunnel: [_ _ _ _ w1054] -> w233
      tunnel: w224 -> [_ _ _ w352 _]
      tunnel: w232 -> [_ _ _ w351 _]
      tunnel: w231 -> [_ _ _ w348 _]
      tunnel: w230 -> [_ _ _ w347 _]
      tunnel: w229 -> [_ _ _ w346 _]
      tunnel: w228 -> [_ _ _ w345 _]
      tunnel: [_ _ _ w344 _] -> w227
      tunnel: w220 -> [_ _ _ w338 _]
      tunnel: w219 -> [_ _ _ w343 _]
      tunnel: [_ _ _ w342 _] -> w226
      tunnel: w225 -> [_ _ _ w341 _]
      tunnel: w224 -> [_ _ _ w340 _]
      tunnel: w222 -> [_ _ _ w339 _]
      tunnel: w220 -> [_ _ _ w337 _]
      tunnel: w218 -> [_ _ _ w336 _]
      tunnel: w216 -> [_ _ _ w335 _]
      tunnel: w215 -> [_ _ _ w334 _]
      tunnel: w214 -> [_ _ _ w333 _]
      tunnel: w212 -> [_ _ _ w332 _]
      frame #0 {
        n109 = while {
          stop <- TRUE stop-if-true
          n110 = Wait (ms)(milliseconds to wait=u32 250) -> ()  [unwired: 1 out]
        }
        n111 = local read "port number 2"() -> (w240:refnum<visa-resource-name>)
        n112 = local read "port number"() -> (w243:refnum<visa-resource-name>)
        n113 = property class="Instr"(reference=w243, "General Settings:Timeout Value"=u32 0) -> (reference out=w242:refnum<visa-resource-name>)  [unwired: 1 in, 1 out]
        n114 = property class="Instr"(reference=w240, "General Settings:Timeout Value"=u32 0) -> (reference out=w239:refnum<visa-resource-name>)  [unwired: 1 in, 1 out]
        n115 = VISA Unlock(11:w242) -> (3:w238:refnum<visa-resource-name>)  [unwired: 1 in, 1 out]
        n116 = VISA Unlock(11:w239) -> (3:w245:refnum<visa-resource-name>)  [unwired: 1 in, 1 out]
        n117 = VISA Close(VISA resource name=w238) -> (error out=→"CLOSE COMMFEM":errorcluster)  [unwired: 1 in]
        n118 = VISA Close(VISA resource name=w245) -> (error out=→"CLOSE COMMBOL":errorcluster)  [unwired: 1 in]
        n119 = while {
          stop <- TRUE stop-if-true
          n120 = Wait (ms)(milliseconds to wait=u32 250) -> ()  [unwired: 1 out]
        }
      }
      frame #1 {
        w261 = T5 0 items=["no dialog", "OK message", "continue or stop message", "OK message + warnings", "continue/stop + warnings"] ("type of dialog (OK msg:1)")
        w265 = T5 0 items=["no dialog", "OK message", "continue or stop message", "OK message + warnings", "continue/stop + warnings"] ("type of dialog (OK msg:1)")
        n121 = call-poly "VISA Configure Serial Port"("VISA resource name"="port number", "termination char\n(0xA = '\\n' = LF)"=enum16{"1 bit", "1.5 bits", "2 bits"}."1 bit" ("stop bits"), "baud rate (9600)"="baud rate", "data bits (8)"="data bit", "parity (0:none)"="parity") -> ("VISA resource name out"=w262:refnum<visa-resource-name>, "error out"=w259:errorcluster)  [unwired: 9 in]
        n122 = Equal?(x="COMMBOL ON_OFF", y="ON") -> (x = y?=w256:bool)
        "BOL OUT" <- w256
        n123 = case shown="True" w256 {
          tunnel: [_ w267] -> w255
          tunnel: [_ w266] -> w254
          frame False {
          }
          frame True {
            n124 = VISA Close(VISA resource name="port number 2") -> (error out=w272:errorcluster)  [unwired: 1 in]
            n125 = call-poly "VISA Configure Serial Port"("VISA resource name"="port number 2", "termination char\n(0xA = '\\n' = LF)"=enum16{"1 bit", "1.5 bits", "2 bits"}."1 bit" ("stop bits"), "baud rate (9600)"="baud rate 2", "data bits (8)"="data bit 2", "parity (0:none)"="parity 2", "error in (no error)"=w272) -> ("VISA resource name out"=w266:refnum<visa-resource-name>, "error out"=w267:errorcluster)  [unwired: 8 in]
          }
        }
        n126 = call <vilib>:"Simple Error Handler.vi"("type of dialog (OK msg:1)"=w261, "error in (no error)"=w255) -> ("message"=w260:string)  [unwired: 3 in, 4 out]
        n127 = call <vilib>:"Simple Error Handler.vi"("type of dialog (OK msg:1)"=w265, "error in (no error)"=w259) -> ("message"=w264:string)  [unwired: 3 in, 4 out]
        n128 = local write "COM err msg: 2"(w260) -> ()
        n129 = local write "COM err msg:"(w264) -> ()
      }
      frame #2 {
        n130 = case shown="No Error" w277 {
          tunnel: w276 -> [w305 _]
          frame No Error {
            n131 = while {
              tunnel: w305 -> [w311]
              stop <- w308 stop-if-true
              n132 = local read "Boolean"() -> (w307:bool)
              n133 = case shown="False" w307 {
                tunnel: w311 -> [w315 _]
                tunnel: [w312 TRUE] -> w309
                frame False {
                  n134 = property class="Instr"(reference=w315) -> (error out=w313:errorcluster, "Serial Settings:Number of Bytes at Serial Port"=w314:u32)  [unwired: 1 in, 1 out]
                  n135 = Greater Than 0?(x=w314) -> (x > 0?=w316:bool)
                  n136 = case shown="True" w316 {
                    selector: w316 -> [w317 _]
                    tunnel: w315 -> [_ w330]
                    tunnel: w314 -> [_ w329]
                    tunnel: w313 -> [_ w328]
                    tunnel: [w317 w319] -> w312
                    frame False {
                    }
                    frame True {
                      n137 = VISA Read(VISA resource name=w330, byte count=w329, error in (no error)=w328) -> (read buffer=w322:string, error out=w325:errorcluster)  [unwired: 2 out]
                      n138 = local write "data string FEM"(w322) -> ()
                      n139 = Unbundle By Name(w325) -> ("status"=w324:bool)
                      n140 = Concatenate Strings("r " ("string"), "\r") -> (w323:string)
                      n141 = Match Pattern(string=w322, regular expression=w323) -> (offset past match=w321:i32)  [unwired: 1 in, 3 out]
                      n142 = Not Equal?(x=w321, y=-1) -> (x != y?=w318:bool)
                      "Boolean" <- w318
                      n143 = Or(x=w318, y=w324) -> (x .or. y?=w319:bool)
                    }
                  }
                }
                frame True {
                }
              }
              n144 = Wait (ms)(milliseconds to wait=u32 1000) -> ()  [unwired: 1 out]
              n145 = Or(x=w309, y=TRUE) -> (x .or. y?=w308:bool)
            }
          }
          frame Error {
          }
        }
        n146 = case shown="No Error" w274 {
          tunnel: w275 -> [w278 _]
          frame No Error {
            n147 = while {
              tunnel: w278 -> [w284]
              stop <- w281 stop-if-true
              n148 = local read "Boolean 2"() -> (w279:bool)
              n149 = case shown="False" w279 {
                tunnel: w284 -> [w288 _]
                tunnel: [w285 TRUE] -> w282
                frame False {
                  n150 = property class="Instr"(reference=w288) -> (error out=w286:errorcluster, "Serial Settings:Number of Bytes at Serial Port"=w287:u32)  [unwired: 1 in, 1 out]
                  n151 = Greater Than 0?(x=w287) -> (x > 0?=w289:bool)
                  n152 = case shown="True" w289 {
                    selector: w289 -> [w290 _]
                    tunnel: w288 -> [_ w303]
                    tunnel: w287 -> [_ w302]
                    tunnel: w286 -> [_ w301]
                    tunnel: [w290 w292] -> w285
                    frame False {
                    }
                    frame True {
                      n153 = VISA Read(VISA resource name=w303, byte count=w302, error in (no error)=w301) -> (read buffer=w295:string, error out=w298:errorcluster)  [unwired: 2 out]
                      n154 = local write "data string 3"(w295) -> ()
                      n155 = Unbundle By Name(w298) -> ("status"=w297:bool)
                      n156 = Concatenate Strings("r " ("string"), "\r") -> (w296:string)
                      n157 = Match Pattern(string=w295, regular expression=w296) -> (offset past match=w294:i32)  [unwired: 1 in, 3 out]
                      n158 = Not Equal?(x=w294, y=-1) -> (x != y?=w291:bool)
                      "Boolean 2" <- w291
                      n159 = Or(x=w291, y=w297) -> (x .or. y?=w292:bool)
                    }
                  }
                }
                frame True {
                }
              }
              n160 = Wait (ms)(milliseconds to wait=u32 1000) -> ()  [unwired: 1 out]
              n161 = Or(x=w282, y=TRUE) -> (x .or. y?=w281:bool)
            }
          }
          frame Error {
          }
        }
      }
      frame #3 {
        n162 = case shown="No Error" w350 {
          tunnel: w350 -> [w380 _]
          tunnel: w354 -> [_ w419]
          tunnel: w351 -> [_ w418]
          tunnel: w348 -> [_ w417]
          tunnel: w347 -> [_ w416]
          tunnel: w346 -> [_ w407]
          tunnel: [w379 w395] -> w344
          tunnel: w338 -> [w378 w410]
          tunnel: w343 -> [w379 w409]
          tunnel: [w378 w399] -> w342
          tunnel: w341 -> [_ w387]
          tunnel: w340 -> [_ w388]
          tunnel: w339 -> [_ w401]
          tunnel: w337 -> [_ w398]
          tunnel: w336 -> [_ w396]
          tunnel: w335 -> [_ w392]
          tunnel: w334 -> [_ w393]
          tunnel: w333 -> [_ w391]
          tunnel: w332 -> [_ w383]
          frame Error {
            w381 = T5 0 items=["no dialog", "OK message", "continue or stop message", "OK message + warnings", "continue/stop + warnings"] ("type of dialog (OK msg:1)")
            n163 = call <vilib>:"Simple Error Handler.vi"("type of dialog (OK msg:1)"=w381, "error in (no error)"=w380) -> ("message"=w382:string)  [unwired: 3 in, 4 out]
            n164 = local write "COM err msg:"(w382) -> ()
          }
          frame No Error {
            # "LOCATOR_User.txt"
            # "temp.csv"
            # "LOCATOR_User.csv"
            # "Invio dati via FTP"
            # "Calcolo della media"
            n165 = control-ref of="temp.csv midnight"() -> (w394:refnum<vi>)
            n166 = Equal?(x="SOCKET ON_OFF", y="ON") -> (x = y?=w403:bool)
            "SOCKET" <- w403
            n167 = case shown="True" w403 {
              tunnel: "Socket Port" -> [_ w701]
              frame False {
              }
              frame True {
                w700 = T5 0 items=["no dialog", "OK message", "continue or stop message", "OK message + warnings", "continue/stop + warnings"] ("type of dialog (OK msg:1)")
                # "Check for errors\nand reset Stop \nbutton to False."
                # "Inner Case Structure - True Case Sends a \"we're done\" indication and then waits for \"all received\" response.  If it has not received it in 60 seconds, it gives up.  If the user hits the stop button in the listen loop, the Connection Timed Out error will flow through this part of the case and be cleared. False Case sends the data selected from the Function control on the front panel."
                # "Check if there is a local or remote stop request."
                # "Set Port number."
                # "Inner While Loop - Listen for connection at the port specified.  The Error to Warning.vi subVI is used to turn the time out error to a warning.  Loop stops once a connection is determined."
                # "Note: The Error to Warning.vi is used in this VI to set time out errors and End of Connection errors as warnings.  In a VI where you would want these errors to occur and stop your application or perform some other task based on the error you would not use this SubVI."
                # "Convert a possible Connection Closed error from the client to a warning.  Close the client connection (if it existed) and stop the server if requested or an error in the listener occured."
                n168 = while {
                  tunnel: [w710] -> w702
                  tunnel: w701 -> [w716]
                  stop <- w717 continue-if-true
                  w706 = 66 items=["No Error", "Argument Error", "Memory Full", "Out of Zone", "End of File", "File Already Open", "Generic File IO Error", "File Not Found", "File Permission Error", "Disk Full", "Duplicate Path", "Too Many Files Open", "Not Enabled", "Resource File Not Found", "Cannot Add Resource", "Resource Not Found", "Image Not Found", "Image Memory Error", "Pen Does Not Exist", "Config Bad Type", "Config Token Not Found", "Config Parse Error", "Config Memory Error", "Bad External Code Format", "Bad External Code Offset", "External Code Not Present", "Null Window", "Destroy Window Mixup", "Null Menu", "Print Aborted", "Bad Print Record", "Print Driver Error", "Windows Error During Print", "Memory Error During Print", "Print Dialog Error", "Generic Print Error", "Invalid Device Refnum", "Device Not Found", "Device Parameter Error", "Device Unit Error", "Can't Open Device", "Device Call Aborted", "Generic Error", "Cancelled By User", "Object ID Too Low", "Object ID Too High", "Object Not In Heap", "Unknown Heap", "Bad DefProc ID", "DefProc Not In Table", "Message Out Of Range", "Null Method", "Unknown Message", "Manager Call Not Supported", "Bad address", "Connection In progress", "Connection timed out", "Connection is already in progress", "Network attribute not supported", "Network error", "Address in use", "System out of memory", "Connection aborted", "Connection refused", "Connection is not connected", "Connection is already connected", "Connection closed", "Initialize error (interapplication manager)", "Bad occurrence", "Wait on unbound occurrence handler", "Occurrence queue overflow", "Bad path", "Semaphore not signaled", "Unrecognized type (interapplication manager)"] ("2nd Error to Convert")
                  w707 = 64 items=["No Error", "Argument Error", "Memory Full", "Out of Zone", "End of File", "File Already Open", "Generic File IO Error", "File Not Found", "File Permission Error", "Disk Full", "Duplicate Path", "Too Many Files Open", "Not Enabled", "Resource File Not Found", "Cannot Add Resource", "Resource Not Found", "Image Not Found", "Image Memory Error", "Pen Does Not Exist", "Config Bad Type", "Config Token Not Found", "Config Parse Error", "Config Memory Error", "Bad External Code Format", "Bad External Code Offset", "External Code Not Present", "Null Window", "Destroy Window Mixup", "Null Menu", "Print Aborted", "Bad Print Record", "Print Driver Error", "Windows Error During Print", "Memory Error During Print", "Print Dialog Error", "Generic Print Error", "Invalid Device Refnum", "Device Not Found", "Device Parameter Error", "Device Unit Error", "Can't Open Device", "Device Call Aborted", "Generic Error", "Cancelled By User", "Object ID Too Low", "Object ID Too High", "Object Not In Heap", "Unknown Heap", "Bad DefProc ID", "DefProc Not In Table", "Message Out Of Range", "Null Method", "Unknown Message", "Manager Call Not Supported", "Bad address", "Connection In progress", "Connection timed out", "Connection is already in progress", "Network attribute not supported", "Network error", "Address in use", "System out of memory", "Connection aborted", "Connection refused", "Connection is not connected", "Connection is already connected", "Connection closed", "Initialize error (interapplication manager)", "Bad occurrence", "Wait on unbound occurrence handler", "Occurrence queue overflow", "Bad path", "Semaphore not signaled", "Unrecognized type (interapplication manager)"] ("1st Error to Convert")
                  n169 = while {
                    tunnel: [w718] -> w713
                    tunnel: [w727] -> w714
                    tunnel: [w731] -> w715
                    tunnel: w716 -> [w732]
                    stop <- w729 continue-if-true
                    w718 = FALSE
                    w725 = 56 items=["No Error", "Argument Error", "Memory Full", "Out of Zone", "End of File", "File Already Open", "Generic File IO Error", "File Not Found", "File Permission Error", "Disk Full", "Duplicate Path", "Too Many Files Open", "Not Enabled", "Resource File Not Found", "Cannot Add Resource", "Resource Not Found", "Image Not Found", "Image Memory Error", "Pen Does Not Exist", "Config Bad Type", "Config Token Not Found", "Config Parse Error", "Config Memory Error", "Bad External Code Format", "Bad External Code Offset", "External Code Not Present", "Null Window", "Destroy Window Mixup", "Null Menu", "Print Aborted", "Bad Print Record", "Print Driver Error", "Windows Error During Print", "Memory Error During Print", "Print Dialog Error", "Generic Print Error", "Invalid Device Refnum", "Device Not Found", "Device Parameter Error", "Device Unit Error", "Can't Open Device", "Device Call Aborted", "Generic Error", "Cancelled By User", "Object ID Too Low", "Object ID Too High", "Object Not In Heap", "Unknown Heap", "Bad DefProc ID", "DefProc Not In Table", "Message Out Of Range", "Null Method", "Unknown Message", "Manager Call Not Supported", "Bad address", "Connection In progress", "Connection timed out", "Connection is already in progress", "Network attribute not supported", "Network error", "Address in use", "System out of memory", "Connection aborted", "Connection refused", "Connection is not connected", "Connection is already connected", "Connection closed", "Initialize error (interapplication manager)", "Bad occurrence", "Wait on unbound occurrence handler", "Occurrence queue overflow", "Bad path", "Semaphore not signaled", "Unrecognized type (interapplication manager)"] ("1st Error to Convert")
                    w726 = 56 items=["No Error", "Argument Error", "Memory Full", "Out of Zone", "End of File", "File Already Open", "Generic File IO Error", "File Not Found", "File Permission Error", "Disk Full", "Duplicate Path", "Too Many Files Open", "Not Enabled", "Resource File Not Found", "Cannot Add Resource", "Resource Not Found", "Image Not Found", "Image Memory Error", "Pen Does Not Exist", "Config Bad Type", "Config Token Not Found", "Config Parse Error", "Config Memory Error", "Bad External Code Format", "Bad External Code Offset", "External Code Not Present", "Null Window", "Destroy Window Mixup", "Null Menu", "Print Aborted", "Bad Print Record", "Print Driver Error", "Windows Error During Print", "Memory Error During Print", "Print Dialog Error", "Generic Print Error", "Invalid Device Refnum", "Device Not Found", "Device Parameter Error", "Device Unit Error", "Can't Open Device", "Device Call Aborted", "Generic Error", "Cancelled By User", "Object ID Too Low", "Object ID Too High", "Object Not In Heap", "Unknown Heap", "Bad DefProc ID", "DefProc Not In Table", "Message Out Of Range", "Null Method", "Unknown Message", "Manager Call Not Supported", "Bad address", "Connection In progress", "Connection timed out", "Connection is already in progress", "Network attribute not supported", "Network error", "Address in use", "System out of memory", "Connection aborted", "Connection refused", "Connection is not connected", "Connection is already connected", "Connection closed", "Initialize error (interapplication manager)", "Bad occurrence", "Wait on unbound occurrence handler", "Occurrence queue overflow", "Bad path", "Semaphore not signaled", "Unrecognized type (interapplication manager)"] ("1st Error to Convert")
                    n170 = call <vilib>:"TCP Listen.vi"("timeout ms (wait forever: -1)"=5000, "port"=w732) -> ("error out"=w728:errorcluster, "connection ID"=w731:refnum<k5>)  [unwired: 6 in, 2 out]
                    n171 = Unbundle(w728) -> ("status"=w723:bool, "code"=w724:i32)  [unwired: 1 out]
                    n172 = Not Equal?(x=w724, y=w725) -> (x != y?=w722:bool)
                    n173 = Not(x=w723) -> (.not. x?=w721:bool)
                    n174 = And(x=w723, y=w722) -> (x .and. y?=w720:bool)
                    n175 = Or(x=w721, y=w720) -> (x .or. y?=w719:bool)
                    n176 = call <vilib>:"Error to Warning.vi"("1st Error to Convert"=w726, "error in"=w728) -> ("warning out"=w727:errorcluster)  [unwired: 13 in]
                    n177 = Not Or(1:w719, 2:w718) -> (0:w729:bool)
                  }
                  n178 = Wait (ms)(milliseconds to wait=u32 2000) -> ()  [unwired: 1 out]
                  n179 = case shown="False" w713 {
                    selector: w713 -> [_ w778]
                    tunnel: [w737 w779] -> w705
                    tunnel: w715 -> [w736 w780]
                    tunnel: w714 -> [w735 w779]
                    tunnel: [w734 w780] -> w712
                    tunnel: [w733 w778] -> w708
                    frame False {
                      n180 = while {
                        tunnel: [w738] -> w733
                        tunnel: w735 -> [w753]
                        tunnel: [w744] -> w737
                        tunnel: [w749] -> w734
                        tunnel: w736 -> [w752]
                        stop <- w756 continue-if-true
                        w738 = FALSE
                        w742 = 56 items=["No Error", "Argument Error", "Memory Full", "Out of Zone", "End of File", "File Already Open", "Generic File IO Error", "File Not Found", "File Permission Error", "Disk Full", "Duplicate Path", "Too Many Files Open", "Not Enabled", "Resource File Not Found", "Cannot Add Resource", "Resource Not Found", "Image Not Found", "Image Memory Error", "Pen Does Not Exist", "Config Bad Type", "Config Token Not Found", "Config Parse Error", "Config Memory Error", "Bad External Code Format", "Bad External Code Offset", "External Code Not Present", "Null Window", "Destroy Window Mixup", "Null Menu", "Print Aborted", "Bad Print Record", "Print Driver Error", "Windows Error During Print", "Memory Error During Print", "Print Dialog Error", "Generic Print Error", "Invalid Device Refnum", "Device Not Found", "Device Parameter Error", "Device Unit Error", "Can't Open Device", "Device Call Aborted", "Generic Error", "Cancelled By User", "Object ID Too Low", "Object ID Too High", "Object Not In Heap", "Unknown Heap", "Bad DefProc ID", "DefProc Not In Table", "Message Out Of Range", "Null Method", "Unknown Message", "Manager Call Not Supported", "Bad address", "Connection In progress", "Connection timed out", "Connection is already in progress", "Network attribute not supported", "Network error", "Address in use", "System out of memory", "Connection aborted", "Connection refused", "Connection is not connected", "Connection is already connected", "Connection closed", "Initialize error (interapplication manager)", "Bad occurrence", "Wait on unbound occurrence handler", "Occurrence queue overflow", "Bad path", "Semaphore not signaled", "Unrecognized type (interapplication manager)"] ("1st Error to Convert")
                        n181 = TCP Read(connection ID=w752, bytes to read=1, error in (no error)=w753, 9:0) -> (connection ID out=w750:refnum<k5>, data out=w751:string, error out=w741:errorcluster)  [unwired: 1 in]
                        n182 = Wait (ms)(milliseconds to wait=u32 2000) -> ()  [unwired: 1 out]
                        n183 = String Length(string=w751) -> (length=w747:i32)
                        n184 = Not Equal To 0?(x=w747) -> (x != 0?=w746:bool)
                        n185 = Or(x=w738, y=w746) -> (x .or. y?=w745:bool)
                        n186 = call <vilib>:"Error to Warning.vi"("1st Error to Convert"=w742, "error in"=w741) -> ("warning out"=w740:errorcluster)  [unwired: 13 in]
                        n187 = case shown="False" w745 {
                          tunnel: w740 -> [w758 w773]
                          tunnel: w750 -> [w759 w771]
                          tunnel: [w763 w775] -> w749
                          tunnel: [w762 w766] -> w744
                          tunnel: [FALSE TRUE] -> w748
                          frame False {
                            n188 = local read "Multi socket String"() -> (w757:string)
                            n189 = Type Cast(x=w757) -> (*(type *) &x=w764:string)  [unwired: 1 in]
                            n190 = TCP Write(connection ID=w759, data in=w764, error in (no error)=w758) -> (connection ID out=w763:refnum<k5>, error out=w762:errorcluster)  [unwired: 1 in, 1 out]
                            n191 = Wait (ms)(milliseconds to wait=u32 25) -> ()  [unwired: 1 out]
                          }
                          frame True {
                            w765 = 56 items=["No Error", "Argument Error", "Memory Full", "Out of Zone", "End of File", "File Already Open", "Generic File IO Error", "File Not Found", "File Permission Error", "Disk Full", "Duplicate Path", "Too Many Files Open", "Not Enabled", "Resource File Not Found", "Cannot Add Resource", "Resource Not Found", "Image Not Found", "Image Memory Error", "Pen Does Not Exist", "Config Bad Type", "Config Token Not Found", "Config Parse Error", "Config Memory Error", "Bad External Code Format", "Bad External Code Offset", "External Code Not Present", "Null Window", "Destroy Window Mixup", "Null Menu", "Print Aborted", "Bad Print Record", "Print Driver Error", "Windows Error During Print", "Memory Error During Print", "Print Dialog Error", "Generic Print Error", "Invalid Device Refnum", "Device Not Found", "Device Parameter Error", "Device Unit Error", "Can't Open Device", "Device Call Aborted", "Generic Error", "Cancelled By User", "Object ID Too Low", "Object ID Too High", "Object Not In Heap", "Unknown Heap", "Bad DefProc ID", "DefProc Not In Table", "Message Out Of Range", "Null Method", "Unknown Message", "Manager Call Not Supported", "Bad address", "Connection In progress", "Connection timed out", "Connection is already in progress", "Network attribute not supported", "Network error", "Address in use", "System out of memory", "Connection aborted", "Connection refused", "Connection is not connected", "Connection is already connected", "Connection closed", "Initialize error (interapplication manager)", "Bad occurrence", "Wait on unbound occurrence handler", "Occurrence queue overflow", "Bad path", "Semaphore not signaled", "Unrecognized type (interapplication manager)"] ("1st Error to Convert")
                            n192 = Type Cast(x=0) -> (*(type *) &x=w768:string)  [unwired: 1 in]
                            n193 = TCP Write(connection ID=w771, data in=w768, error in (no error)=w773) -> (connection ID out=w770:refnum<k5>, error out=w772:errorcluster)  [unwired: 1 in, 1 out]
                            n194 = TCP Read(connection ID=w770, bytes to read=1, error in (no error)=w772, 9:60000) -> (connection ID out=w775:refnum<k5>, error out=w767:errorcluster)  [unwired: 1 in, 1 out]
                            n195 = call <vilib>:"Error to Warning.vi"("1st Error to Convert"=w765, "error in"=w767) -> ("warning out"=w766:errorcluster)  [unwired: 13 in]
                          }
                        }
                        n196 = Unbundle By Name(w744) -> ("status"=w743:bool)
                        n197 = Not Or(1:w748, 2:w743) -> (0:w756:bool)
                      }
                    }
                    frame True {
                    }
                  }
                  n198 = call <vilib>:"Error to Warning.vi"("1st Error to Convert"=w707, "2nd Error to Convert"=w706, "error in"=w705) -> ("warning out"=w704:errorcluster)  [unwired: 12 in]
                  n199 = Not A Number/Path/Refnum?(number/path/refnum=w712) -> (NaN/Path/Refnum?=w711:bool)
                  n200 = case shown="False" w711 {
                    tunnel: w704 -> [w783 w784]
                    tunnel: w712 -> [w782 _]
                    tunnel: [w781 w784] -> w710
                    frame False {
                      n201 = TCP Close Connection(connection ID=w782, error in (no error)=w783) -> (error out=w781:errorcluster)  [unwired: 1 in, 1 out]
                    }
                    frame True {
                    }
                  }
                  n202 = Unbundle By Name(w710) -> ("status"=w709:bool)
                  n203 = Not Or(1:w709, 2:w708) -> (0:w717:bool)
                }
                n204 = call <vilib>:"General Error Handler.vi"("type of dialog (OK msg:1)"=w700, "error in (no error)"=w702) -> ()  [unwired: 9 in, 5 out]
              }
            }
            n205 = control-ref of="FTP"() -> (w415:refnum<vi>)
            n206 = while {
              stop <- TRUE continue-if-true
              n207 = property on="In allarme VHf ?" class="Bool (strict)"() -> ("Value"=w672:bool)  [unwired: 2 in, 2 out]
              "In ripetizione VHf ?" <- w672
              n208 = case shown="True" w672 {
                frame False {
                  n209 = property on="Numero ripetizioni alarm VHf" class="DigNum (strict)"("Value"=0) -> ()  [unwired: 2 in, 2 out]
                  n210 = property on="Ripetizioni alarm VHf" class="Bool (strict)"("Value"=FALSE) -> ()  [unwired: 2 in, 2 out]
                }
                frame True {
                  # "Ciclo temporizzazione\nallarme Very High Field"
                  n211 = property on="Seconds Very High field alarm" class="DigNum (strict)"() -> ("Value"=w677:sgl)  [unwired: 2 in, 2 out]
                  n212 = Multiply(x=w677, y=4) -> (x*y=w675:sgl)
                  n213 = property on="Numero ripetizioni alarm VHf" class="DigNum (strict)"("Value"=w675) -> ()  [unwired: 2 in, 2 out]
                  n214 = while {
                    i -> [w680]
                    stop <- w682 stop-if-true
                    n215 = Less Or Equal?(x="Numero ripetizioni alarm VHf", y=w680) -> (x <= y?=w682:bool)
                    n216 = property on="Ripetizioni alarm VHf" class="Bool (strict)"("Value"=TRUE) -> ()  [unwired: 2 in, 2 out]
                    n217 = Wait Until Next ms Multiple(millisecond multiple=250) -> ()  [unwired: 1 out]
                    n218 = property on="Numero ripetizioni alarm Hf" class="DigNum (strict)"("Value"=0) -> ()  [unwired: 2 in, 2 out]
                    "Alarm VHf counter" <- w680
                  }
                }
              }
              n219 = Wait Until Next ms Multiple(millisecond multiple=250) -> ()  [unwired: 1 out]
            }
            n220 = while {
              stop <- TRUE continue-if-true
              n221 = property on="In allarme Hf ?" class="Bool (strict)"() -> ("Value"=w687:bool)  [unwired: 2 in, 2 out]
              n222 = property on="In ripetizione VHf ?" class="Bool (strict)"() -> ("Value"=w684:bool)  [unwired: 2 in, 2 out]
              n223 = Implies(1:w684, 2:w687) -> (0:w686:bool)
              n224 = Not(x=w686) -> (.not. x?=w685:bool)
              n225 = case shown="True" w685 {
                frame False {
                  n226 = property on="Numero ripetizioni alarm Hf" class="DigNum (strict)"("Value"=0) -> ()  [unwired: 2 in, 2 out]
                  n227 = property on="Ripetizioni alarm Hf" class="Bool (strict)"("Value"=FALSE) -> ()  [unwired: 2 in, 2 out]
                }
                frame True {
                  # "Ciclo temporizzazione\nallarme High Field"
                  n228 = property on="Seconds High field alarm" class="DigNum (strict)"() -> ("Value"=w694:sgl)  [unwired: 2 in, 2 out]
                  n229 = Multiply(x=w694, y=4) -> (x*y=w692:sgl)
                  n230 = property on="Numero ripetizioni alarm Hf" class="DigNum (strict)"("Value"=w692) -> ()  [unwired: 2 in, 2 out]
                  n231 = while {
                    i -> [w697]
                    stop <- w696 stop-if-true
                    n232 = Less Or Equal?(x="Numero ripetizioni alarm Hf", y=w697) -> (x <= y?=w696:bool)
                    n233 = Wait Until Next ms Multiple(millisecond multiple=250) -> ()  [unwired: 1 out]
                    n234 = property on="Ripetizioni alarm Hf" class="Bool (strict)"("Value"=TRUE) -> ()  [unwired: 2 in, 2 out]
                    "Alarm Hf counter" <- w697
                  }
                }
              }
              n235 = Wait Until Next ms Multiple(millisecond multiple=250) -> ()  [unwired: 1 out]
            }
            n236 = node-c288() -> (w389:T2)  [unwired: 1 in]
            n237 = call "Mediated_Values.vi"("coda kV/m mediati"=w407, "coda mV"=w416) -> ("4 valori per media\nin array"=→"4 valori per media in array":dbl[])  [unwired: 1 in, 2 out]
            n238 = timed-loop {
              timing-out: [_] -> w390
              timing: w389 -> [_]
              stop <- TRUE continue-if-true
              w473 = u8 6 ("X Scale.Style")
              w488 = u32 0
              w489 = u32 0
              w491 = u32 0
              w493 = u32 0
              w528 = u32 0
              w517 = TRUE
              w541 = 60
              w551 = u32 0
              w518 = TRUE
              w568 = 60
              w578 = u32 0
              w519 = TRUE
              w595 = 60
              w610 = 60
              w525 = u32 0
              w520 = TRUE
              # "Creazione del nome del file\ndell'immagine giornaliera"
              # "Creazione delle stringhe da\ninserire sul grafico"
              # "Creazione del grafico 24 ore"
              # "Secondi a partire dalla mezzanotte"
              # "Creazione del grafico 4 ore"
              # "Secondi a partire dalla mezzanotte"
              # "Creazione del grafico 1 ora"
              # "Secondi a partire dalla mezzanotte"
              # "Secondi a partire dalla mezzanotte"
              # "Creazione del grafico corrente"
              n239 = node-c288() -> ()  [unwired: 1 in, 2 out]
              n240 = Get Date/Time In Seconds() -> (seconds since 1Jan1904=w467:timestamp)
              n241 = Get Date/Time In Seconds() -> (seconds since 1Jan1904=w468:timestamp)
              n242 = Get Date/Time In Seconds() -> (seconds since 1Jan1904=w466:timestamp)
              n243 = Get Date/Time In Seconds() -> (seconds since 1Jan1904=w469:timestamp)
              n244 = control-ref of="FEM software v.2.4 - Live Graph"() -> ()  [unwired: 1 out]
              n245 = call <vilib>:"LV70TimeStampToDateRec.vi"("time stamp"=w467) -> ("date time rec"=w599:T6)
              n246 = call <vilib>:"LV70TimeStampToDateRec.vi"("time stamp"=w468) -> ("date time rec"=w572:T6)
              n247 = call <vilib>:"LV70TimeStampToDateRec.vi"("time stamp"=w466) -> ("date time rec"=w614:T6)
              n248 = call <vilib>:"LV70TimeStampToDateRec.vi"("time stamp"=w469) -> ("date time rec"=w545:T6)
              n249 = Get Date/Time In Seconds() -> (seconds since 1Jan1904=w482:timestamp)
              n250 = Unbundle By Name(w599) -> ("second"=w592:i32, "minute"=w593:i32, "hour"=w598:i32)
              n251 = Unbundle By Name(w572) -> ("second"=w565:i32, "minute"=w566:i32, "hour"=w571:i32)
              n252 = Unbundle By Name(w614) -> ("second"=w607:i32, "minute"=w608:i32, "hour"=w613:i32)
              n253 = Get Date/Time In Seconds() -> (seconds since 1Jan1904=w515:timestamp)
              n254 = Unbundle By Name(w545) -> ("second"=w538:i32, "minute"=w539:i32, "hour"=w544:i32)
              n255 = Multiply(x=w598, y=w595) -> (x*y=w597:i32)
              n256 = Multiply(x=w571, y=w568) -> (x*y=w570:i32)
              n257 = Multiply(x=w613, y=w610) -> (x*y=w612:i32)
              n258 = control-ref of="FEM Graph_IMAGES"() -> (w474:refnum<vi>)
              n259 = Multiply(x=w544, y=w541) -> (x*y=w543:i32)
              n260 = Add(x=w593, y=w597) -> (x+y=w596:i32)
              n261 = Add(x=w566, y=w570) -> (x+y=w569:i32)
              n262 = Add(x=w608, y=w612) -> (x+y=w611:i32)
              n263 = Format Date/Time String(time format string (%c)=" %d-%m-%y / %H:%M:%S", seconds (now)=w482) -> (date/time string=w504:string)  [unwired: 1 in]
              n264 = Format Date/Time String(time format string (%c)="%d-%m-%y", seconds (now)=w482) -> (date/time string=w479:string)  [unwired: 1 in]
              n265 = Format Date/Time String(time format string (%c)=" %d-%m-%y / %H:%M:%S", seconds (now)=w515) -> (date/time string=w514:string)  [unwired: 1 in]
              n266 = Add(x=w539, y=w543) -> (x+y=w542:i32)
              n267 = Multiply(x=w596, y=w595) -> (x*y=w594:i32)
              n268 = Multiply(x=w569, y=w568) -> (x*y=w567:i32)
              n269 = Multiply(x=w611, y=w610) -> (x*y=w609:i32)
              n270 = Multiply(x=w542, y=w541) -> (x*y=w540:i32)
              n271 = Strip Path(path="Path24hourFile") -> (stripped path=w483:path)  [unwired: 1 out]
              n272 = Add(x=w592, y=w594) -> (x+y=w591:i32)
              n273 = Add(x=w565, y=w567) -> (x+y=w564:i32)
              n274 = Add(x=w607, y=w609) -> (x+y=w606:i32)
              n275 = Add(x=w538, y=w540) -> (x+y=w537:i32)
              n276 = Concatenate Strings("FEM_", w479, ".jpg") -> (w477:string)
              n277 = Subtract(x=w591, y=w595) -> (x-y=w600:i32)
              n278 = Subtract(x=w564, y=w568) -> (x-y=w573:i32)
              n279 = Subtract(x=w606, y=w610) -> (x-y=w615:i32)
              n280 = Add(x=sgl 0.0, y=w600) -> (x+y=w588:sgl)
              n281 = Add(x=sgl 0.0, y=w573) -> (x+y=w561:sgl)
              n282 = Add(x=sgl 0.0, y=w615) -> (x+y=w604:sgl)
              n283 = Subtract(x=w537, y=w541) -> (x-y=w546:i32)
              n284 = Add(x=sgl 0.0, y=w546) -> (x+y=w471:sgl)
              n285 = Build Path(base path=w483, name or relative path=w477) -> (appended path=w476:path)
              n286 = local read "LiveGraph string"() -> (w511:string)
              n287 = local read "24hour graph string"() -> (w494:string)
              n288 = local read "1hour graph string"() -> (w496:string)
              n289 = property on="Property Node" class="XYGraph (strict)"(reference=w474, "X Scale.Range:Minimum"=300.0, "X Scale.Range:Maximum"=w471, "X Scale.Range:Increment"=w471, "X Scale.Style"=w473) -> (reference out=w526:refnum<vi>)  [unwired: 1 in, 1 out]
              n290 = Subtract(x=w588, y=3600) -> (x-y=w589:sgl)
              n291 = property on="Property Node" class="XYGraph (strict)"(reference=w474, "X Scale.Range:Minimum"=w589, "X Scale.Range:Maximum"=w588, "X Scale.Range:Increment"=w588, "X Scale.Style"=w473) -> (reference out=w576:refnum<vi>)  [unwired: 1 in, 1 out]
              n292 = Subtract(x=w561, y=14400) -> (x-y=w562:sgl)
              n293 = property on="Property Node" class="XYGraph (strict)"(reference=w474, "X Scale.Range:Minimum"=w562, "X Scale.Range:Maximum"=w561, "X Scale.Range:Increment"=w561, "X Scale.Style"=w473) -> (reference out=w549:refnum<vi>)  [unwired: 1 in, 1 out]
              n294 = Subtract(x=w604, y=320) -> (x-y=w605:sgl)
              n295 = property on="Property Node" class="XYGraph (strict)"(reference=w474, "X Scale.Range:Minimum"=w605, "X Scale.Range:Maximum"=w604, "X Scale.Range:Increment"=w604, "X Scale.Style"=w473) -> (reference out=w602:refnum<vi>)  [unwired: 1 in, 1 out]
              n296 = local read "4hour graph string"() -> (w495:string)
              n297 = property on="Property Node" class="XYGraph (strict)"(reference=w602, "Palette:Visible"=FALSE, "X Scrollbar Visible"=FALSE, "Caption.Visible"=w520, "Caption.Colors:FG Color"=w525, "Caption.Colors:BG Color"=w525, "YScale.Maximum"=10.0 ("Y Scale.Range:Maximum"), "YScale.Minimum"=-10.0 ("Y Scale.Range:Minimum"), "Caption.Text"=w511, "Caption.Text Colors:Text Color"=u32 16448250, "Caption.Font:Bold"=w520) -> (reference out=w617:refnum<vi>)  [unwired: 1 in, 1 out]
              n298 = Get Date/Time In Seconds() -> (seconds since 1Jan1904=w500:timestamp)
              n299 = Get Date/Time In Seconds() -> (seconds since 1Jan1904=w509:timestamp)
              n300 = property on="Property Node" class="XYGraph (strict)"(reference=w576, "Palette:Visible"=FALSE, "X Scrollbar Visible"=FALSE, "Caption.Visible"=w519, "Caption.Colors:FG Color"=w578, "Caption.Colors:BG Color"=w578, "YScale.Maximum"=10.0 ("Y Scale.Range:Maximum"), "YScale.Minimum"=-10.0 ("Y Scale.Range:Minimum"), "Caption.Text"=w496, "Caption.Text Colors:Text Color"=u32 16448250, "Caption.Font:Bold"=w519) -> (reference out=w577:refnum<vi>)  [unwired: 1 in, 1 out]
              n301 = property on="Property Node" class="XYGraph (strict)"(reference=w549, "Palette:Visible"=FALSE, "X Scrollbar Visible"=FALSE, "Caption.Visible"=w518, "Caption.Colors:FG Color"=w551, "Caption.Colors:BG Color"=w551, "YScale.Maximum"=10.0 ("Y Scale.Range:Maximum"), "YScale.Minimum"=-10.0 ("Y Scale.Range:Minimum"), "Caption.Text"=w495, "Caption.Text Colors:Text Color"=u32 16448250, "Caption.Font:Bold"=w518) -> (reference out=w550:refnum<vi>)  [unwired: 1 in, 1 out]
              n302 = property on="Property Node" class="XYGraph (strict)"(reference=w526, "Palette:Visible"=FALSE, "X Scrollbar Visible"=FALSE, "Caption.Visible"=w517, "Caption.Colors:FG Color"=w528, "Caption.Colors:BG Color"=w528, "YScale.Maximum"=10.0 ("Y Scale.Range:Maximum"), "YScale.Minimum"=-10.0 ("Y Scale.Range:Minimum"), "Caption.Text"=w494, "Caption.Text Colors:Text Color"=u32 16448250, "Caption.Font:Bold"=w517) -> (reference out=w527:refnum<vi>)  [unwired: 1 in, 1 out]
              n303 = Format Date/Time String(time format string (%c)=" %d-%m-%y / %H:%M:%S", seconds (now)=w500) -> (date/time string=w499:string)  [unwired: 1 in]
              n304 = Format Date/Time String(time format string (%c)=" %d-%m-%y / %H:%M:%S", seconds (now)=w509) -> (date/time string=w508:string)  [unwired: 1 in]
              n305 = invoke on="Invoke Node" class="XYGraph (strict)" method="Get Image"(reference=w617, "image depth"=8, "bg color"=u32 0) -> (reference out=w628:refnum<vi>, "image data"=w627:T7)  [unwired: 3 in, 4 out]
              n306 = invoke on="Invoke Node" class="XYGraph (strict)" method="Get Image"(reference=w577, "image depth"=8, "bg color"=u32 0) -> (reference out=w587:refnum<vi>, "image data"=w586:T7)  [unwired: 3 in, 4 out]
              n307 = invoke on="Invoke Node" class="XYGraph (strict)" method="Get Image"(reference=w550, "image depth"=8, "bg color"=u32 0) -> (reference out=w560:refnum<vi>, "image data"=w559:T7)  [unwired: 3 in, 4 out]
              n308 = invoke on="Invoke Node" class="XYGraph (strict)" method="Get Image"(reference=w527, "image depth"=8, "bg color"=u32 0) -> (reference out=w536:refnum<vi>, "image data"=w485:T7)  [unwired: 3 in, 4 out]
              n309 = call <vilib>:"Write JPEG File.vi"("image data"=w627, "path to JPEG file"="PathCurrentFile") -> ()  [unwired: 8 in, 2 out]
              n310 = call <vilib>:"Write JPEG File.vi"("image data"=w586, "path to JPEG file"="Path1hourFile") -> ()  [unwired: 8 in, 2 out]
              n311 = call <vilib>:"Write JPEG File.vi"("image data"=w559, "path to JPEG file"="Path4hourFile") -> ()  [unwired: 8 in, 2 out]
              n312 = call <vilib>:"Write JPEG File.vi"("image data"=w485, "path to JPEG file"="Path24hourFile") -> ()  [unwired: 8 in, 2 out]
              n313 = call <vilib>:"Write JPEG File.vi"("quality (80)"=100, "image data"=w485, "path to JPEG file"=w476) -> ()  [unwired: 7 in, 2 out]
              n314 = property on="Property Node" class="XYGraph (strict)"(reference=w628, "Palette:Visible"=FALSE, "X Scrollbar Visible"=FALSE, "Caption.Visible"=TRUE, "YScale.Maximum"=10.0 ("Y Scale.Range:Maximum"), "YScale.Minimum"=-10.0 ("Y Scale.Range:Minimum"), "Caption.Colors:FG Color"=w493, "Caption.Colors:BG Color"=w493, "Caption.Text Colors:Text Color"=u32 16448250) -> ()  [unwired: 1 in, 2 out]
              n315 = property on="Property Node" class="XYGraph (strict)"(reference=w587, "Palette:Visible"=FALSE, "X Scrollbar Visible"=FALSE, "Caption.Visible"=TRUE, "YScale.Maximum"=10.0 ("Y Scale.Range:Maximum"), "YScale.Minimum"=-10.0 ("Y Scale.Range:Minimum"), "Caption.Colors:FG Color"=w491, "Caption.Colors:BG Color"=w491, "Caption.Text Colors:Text Color"=u32 16448250) -> ()  [unwired: 1 in, 2 out]
              n316 = property on="Property Node" class="XYGraph (strict)"(reference=w560, "Palette:Visible"=FALSE, "X Scrollbar Visible"=FALSE, "Caption.Visible"=TRUE, "YScale.Maximum"=10.0 ("Y Scale.Range:Maximum"), "YScale.Minimum"=-10.0 ("Y Scale.Range:Minimum"), "Caption.Colors:FG Color"=w489, "Caption.Colors:BG Color"=w489, "Caption.Text Colors:Text Color"=u32 16448250) -> ()  [unwired: 1 in, 2 out]
              n317 = local read "Station Info graph"() -> (w472:string)
              n318 = Concatenate Strings("FEM software - 4 hours Graph -", w504, w472) -> (→"4hour graph string":string)
              n319 = Concatenate Strings("FEM software - 5 min Graph -", w514, w472) -> (→"LiveGraph string":string)
              n320 = Concatenate Strings("FEM software - 24 hours Graph -", w499, w472) -> (→"24hour graph string":string)
              n321 = Concatenate Strings("FEM software - 1 hour Graph -", w508, w472) -> (→"1hour graph string":string)
              n322 = property on="Property Node" class="XYGraph (strict)"(reference=w536, "Palette:Visible"=FALSE, "X Scrollbar Visible"=FALSE, "Caption.Visible"=TRUE, "YScale.Maximum"=10.0 ("Y Scale.Range:Maximum"), "YScale.Minimum"=-10.0 ("Y Scale.Range:Minimum"), "Caption.Colors:FG Color"=w488, "Caption.Colors:BG Color"=w488, "Caption.Text Colors:Text Color"=u32 16448250) -> ()  [unwired: 1 in, 2 out]
            }
            n323 = local read "remoteinfopath"() -> (w400:string)
            n324 = call "FTP_file_aktuell.vi"("START_STOP"=w415, "passftp"="passftp", "remotepath"="remotepath", "seconds"="seconds", "temp.csv midnight2"=w394, "ftpsite"="ftpsite", "ref_temp3.csv"=w391, "ref_LOCATOR_User.txt"=w401, "ref_temp.csv"=w398, "ref_LOCATOR_User.csv"=w396, "ref_temp2.csv"=w392, "loginftp"="loginftp", "remoteinfopath"=w400) -> ()  [unwired: 3 in]
            n325 = while {
              tunnel: w419 -> [w997]
              tunnel: w418 -> [w996]
              tunnel: w417 -> [w995]
              stop <- TRUE continue-if-true
              w999 = T5 0 items=["no dialog", "OK message", "continue or stop message", "OK message + warnings", "continue/stop + warnings"] ("type of dialog (OK msg:1)")
              w1002 = u32 500  # Output Rate
              # "Controlla se nel\nfile di configurazione\nè settato il campo\nOFFSET"
              # "Controlla se nel\nfile di configurazione\nè settato il campo\nINVERTED"
              # "MENU ALARMS"
              # "MENU INTERNET"
              # "MENU FILTRI"
              # "Routine principale di lettura dati dalla seriale\ned alcuni filtri.\nIn più controlli per i dati mediati ed invio dati FTP"
              n326 = case shown="True" "About" {
                frame False {
                }
                frame True {
                  n327 = call "MENU_About.vi"() -> ()  [unwired: 6 in]
                }
              }
              n328 = case shown="True" "MENU FILTERS" {
                frame False {
                }
                frame True {
                  n329 = property on="Offset" class="DigNum (strict)"() -> ("Value"=w1051:dbl)  [unwired: 2 in, 2 out]
                  n330 = property on="Inversion sign" class="Bool (strict)"() -> ("Value"=w1053:bool)  [unwired: 2 in, 2 out]
                  n331 = property on="Mediated v." class="Bool (strict)"() -> ("Value"=w1050:bool)  [unwired: 2 in, 2 out]
                  n332 = call "MENU_Filters.vi"("Mediated v."=w1050, "Offset"=w1051, "Inversion sign 2"=w1053) -> ("Mediated v. 2"=→"Mediated v.":bool, "Offset 2"=→"Offset":dbl, "Inversion sign 3"=→"Inversion sign":bool)
                }
              }
              n333 = property class="Instr"(reference=w997) -> (error out=w989:errorcluster, "Serial Settings:Number of Bytes at Serial Port"=w987:u32)  [unwired: 1 in, 1 out]
              n334 = Greater Than 0?(x=w987) -> (x > 0?=w988:bool)
              n335 = Get Date/Time In Seconds() -> (seconds since 1Jan1904=→"Time & Date" →"Time & Date 2":timestamp)
              n336 = case shown="True" "MENU INTERNET" {
                frame False {
                }
                frame True {
                  n337 = property on="FTP" class="Bool (strict)"() -> ("Value"=w1047:bool)  [unwired: 2 in, 2 out]
                  n338 = call "MENU_Internet.vi"("FTP"=w1047) -> ("FTP 2"=→"FTP" →"FTP":bool)  [unwired: 4 in]
                }
              }
              n339 = property on="Inverted_p" class="Str"() -> ("Value"=w983:string)  [unwired: 2 in, 2 out]
              n340 = Not Equal?(x=w983, y="") -> (x != y?=w984:bool)
              n341 = case shown="False" w984 {
                tunnel: [w1005 w1011] -> w982
                frame False {
                  n342 = property on="Inverted_p" class="Str"() -> ("Value"=w1007:string)  [unwired: 2 in, 2 out]
                  n343 = Equal?(x=w1007, y="ON") -> (x = y?=w1006:bool)
                  n344 = case shown="True" w1006 {
                    tunnel: [TRUE FALSE] -> w1005
                    frame False {
                    }
                    frame True {
                    }
                  }
                }
                frame True {
                  n345 = property on="Inversion sign" class="Bool (strict)"() -> ("Value"=w1011:bool)  [unwired: 2 in, 2 out]
                }
              }
              "Inver. sign" <- w982
              n346 = case shown="True" "MENU ALARMS" {
                frame False {
                }
                frame True {
                  n347 = property on="Very High field alarm" class="DigNum (strict)"() -> ("Value"=w1039:sgl)  [unwired: 2 in, 2 out]
                  n348 = property on="High field alarm" class="DigNum (strict)"() -> ("Value"=w1041:sgl)  [unwired: 2 in, 2 out]
                  n349 = property on="Seconds High field alarm" class="DigNum (strict)"() -> ("Value"=w1040:sgl)  [unwired: 2 in, 2 out]
                  n350 = property on="Seconds Very High field alarm" class="DigNum (strict)"() -> ("Value"=w1038:sgl)  [unwired: 2 in, 2 out]
                  n351 = call "MENU_Alarms.vi"("Seconds Very High field alarm"=w1038, "Very High field alarm"=w1039, "Seconds High field alarm"=w1040, "High field alarm"=w1041) -> ("Seconds Very High field alarm 2"=→"Seconds Very High field alarm":sgl, "Very High field alarm 2"=→"Very High field alarm":sgl, "Seconds High field alarm 2"=→"Seconds High field alarm":sgl, "High field alarm 2"=→"High field alarm":sgl)
                }
              }
              n352 = property on="Offset_p" class="DigNum (strict)"() -> ("Value"=w980:i32)  [unwired: 2 in, 2 out]
              n353 = Not Equal To 0?(x=w980) -> (x != 0?=w981:bool)
              n354 = case shown="True" w981 {
                tunnel: [w1003 w1004] -> w979
                frame False {
                  n355 = property on="Offset" class="DigNum (strict)"() -> ("Value"=w1003:dbl)  [unwired: 2 in, 2 out]
                }
                frame True {
                  n356 = property on="Offset_p" class="DigNum (strict)"() -> ("Value"=w1004:i32)  [unwired: 2 in, 2 out]
                }
              }
              "Offset" <- w979
              n357 = case shown="True" w988 {
                tunnel: [w1012 w1027] -> w998
                tunnel: w997 -> [_ w1026]
                tunnel: w987 -> [_ w1025]
                tunnel: w996 -> [_ w1023]
                tunnel: w995 -> [_ w1022]
                tunnel: w989 -> [w1012 w1019]
                tunnel: w982 -> [_ w1018]
                tunnel: w979 -> [_ w1017]
                frame False {
                }
                frame True {
                  # "Coda kV/m"
                  # "Coda mV"
                  # "Filters"
                  n358 = VISA Read(VISA resource name=w1026, byte count=w1025, error in (no error)=w1019) -> (read buffer=w1024:string, error out=w1027:errorcluster)  [unwired: 2 out]
                  "data string FEM" <- w1024
                  n359 = Equal?(x="FEM_ON_OFF", y="ON") -> (x = y?=w1013:bool)
                  n360 = Not(x=w1013) -> (.not. x?=→"BOL IN":bool)
                  n361 = case shown="False" w1013 {
                    tunnel: w1024 -> [w1031 w1037]
                    tunnel: [w1029 w1036] -> w1021
                    tunnel: [w1028 w1035] -> w1020
                    tunnel: w1018 -> [w1030 w1034]
                    tunnel: w1017 -> [w1032 w1033]
                    frame False {
                      n362 = call "BoltekInStr.vi"("Offset"=w1032, "read buffer"=w1031, "controllo_segno"=w1030) -> ("kV/m"=w1028:string, "mV"=w1029:string)
                    }
                    frame True {
                      n363 = call "EFieldInStr.vi"("Offset"=w1033, "read buffer"=w1037, "controllo_segno"=w1034) -> ("kV/m"=w1035:string, "mV"=w1036:string)
                    }
                  }
                  "mV" <- w1021
                  "kV/m" <- w1020
                  n364 = Enqueue Element(queue=w1023, element=w1020) -> ()  [unwired: 2 in, 3 out]
                  n365 = Enqueue Element(queue=w1022, element=w1021) -> ()  [unwired: 2 in, 3 out]
                }
              }
              n366 = Unbundle By Name(w998) -> ("code"=w1001:i32)
              n367 = call <vilib>:"Simple Error Handler.vi"("error code (no error:0)"=w1001, "type of dialog (OK msg:1)"=w999) -> ("message"=→"COM err msg:":string)  [unwired: 3 in, 4 out]
              n368 = Wait (ms)(milliseconds to wait=w1002) -> ()  [unwired: 1 out]
            }
            n369 = while {
              tunnel: w410 -> [w870]
              tunnel: w409 -> [w893]
              tunnel: [w867] -> w399
              tunnel: w387 -> [w892]
              tunnel: w388 -> [w891]
              shift-right: [w875] -> _
              shift-left: string[] [] -> [w872]
              tunnel: [w865] -> w395
              tunnel: w393 -> [w863]
              stop <- TRUE continue-if-true
              w854 = 60
              w789 = ";"
              # "Valutazione degli\nalert da visualizzare\nsul pannello principale"
              # "Controlla se nel\nfile di configurazione\nè settato il campo\nMEDIATED"
              # "Valori Max e Min \nda 1 ora"
              # "Valori Max e Min \nda 10 minuti"
              # "Valori Max e Min \na partire dalla\nmezzanotte"
              # "Controlla che il file graph.txt \nnon sia del giorno prima."
              # "Cancella grafico a mezzanotte:\n3 secondi dopo la mezzanotte"
              # "Secondi a partire dalla mezzanotte"
              # "Questa sezione crea l'Array\nda inviare via socket.\nVedi la stringa qui più sotto."
              # "Controllo la dimensione dell'Array.\nSe è maggiore o uguale di 15 ruota\nl'array altrimenti lo riempie."
              # "Dati per la creazione\ndel grafico"
              # "Questa routine viene richiamata da FTP a mezzanotte per svuotare il file temp.csv e poi viene rimesso in modalità append"
              # "Routine per la scrittura del file temp.csv.\nVisualizzazione e controlli del grafico sul pannello\nprincipale."
              # "Scrittura sul file temp.csv"
              n370 = control-ref of="String Alarm"() -> (w882:refnum<vi>)
              n371 = control-ref of="High field alarm"() -> (w881:refnum<vi>)
              n372 = control-ref of="In ripetizione VHf ?"() -> (w876:refnum<vi>)
              n373 = control-ref of="kV/m tampone"() -> (w805:refnum<vi>)
              n374 = Wait Until Next ms Multiple(millisecond multiple=250) -> ()  [unwired: 1 out]
              n375 = control-ref of="Very High field alarm"() -> (w880:refnum<vi>)
              n376 = Array Size(array=w872) -> (size(s)=w874:i32)
              n377 = control-ref of="kV/m"() -> (w883:refnum<vi>)
              n378 = Greater Or Equal?(x=w874, y=15) -> (x >= y?=w873:bool)
              n379 = Get Date/Time In Seconds() -> (seconds since 1Jan1904=w887:timestamp)
              n380 = property on="Mediated_p" class="Str"() -> ("Value"=w817:string)  [unwired: 2 in, 2 out]
              n381 = Format Date/Time String(time format string (%c)="%H:%M:%S", seconds (now)=w887) -> (date/time string=w890:string)  [unwired: 1 in]
              n382 = Not Equal?(x=w817, y="") -> (x != y?=w815:bool)
              n383 = case shown="True" w815 {
                tunnel: [w913 w915] -> w814
                frame False {
                  n384 = property on="Mediated v." class="Bool (strict)"() -> ("Value"=w913:bool)  [unwired: 2 in, 2 out]
                }
                frame True {
                  n385 = property on="Mediated_p" class="Str"() -> ("Value"=w914:string)  [unwired: 2 in, 2 out]
                  n386 = Equal?(x=w914, y="ON") -> (x = y?=w916:bool)
                  n387 = case shown="True" w916 {
                    tunnel: [FALSE TRUE] -> w915
                    frame False {
                    }
                    frame True {
                    }
                  }
                }
              }
              "Mediated v.." <- w814
              n388 = case shown="False" w814 {
                tunnel: [w975 w977] -> w889
                tunnel: w892 -> [_ w978]
                tunnel: w891 -> [w976 _]
                frame False {
                  # "Coda kV/m"
                  n389 = Dequeue Element(queue=w976) -> ()  [unwired: 2 in, 4 out]
                  n390 = property on="kV/m" class="Str"() -> ("Value"=w975:string)  [unwired: 2 in, 2 out]
                }
                frame True {
                  # "Coda kV/m mediati"
                  n391 = Dequeue Element(queue=w978) -> (element=w977:string)  [unwired: 2 in, 3 out]
                }
              }
              n392 = Fract/Exp String To Number(use system decimal point (T)=FALSE, string=w889) -> (number=w787:dbl)  [unwired: 2 in, 1 out]
              n393 = call "strike_distance.vi"("Numeric"=w787, "reference"=w805) -> ("Strike distance Km"=w785:dbl, "kV/m tampone"=→"kV/m tampone":dbl)
              "Strike distance Km" <- w785
              n394 = Absolute Value(x=w787) -> (abs(x)=w786:dbl)
              n395 = call "Allarmi_High_Low_Field.vi"("Numeric"=w786, "Ripetizioni alarm Hf"="Ripetizioni alarm Hf", "reference 5"=w876, "reference 4"=w880, "reference 3"=w881, "Ripetizioni alarm VHf"="Ripetizioni alarm VHf", "reference 2"=w882, "reference"=w883) -> ("String Alarm"=→"String Alarm":string, "In allarme VHf ?"=→"In allarme VHf ?":bool, "In allarme Hf ?"=→"In allarme Hf ?":bool)
              n396 = Number To Decimal String(number=w785) -> (decimal integer string=w788:string)  [unwired: 1 in]
              n397 = In Range and Coerce(upper limit=40.0, x=w785, lower limit=31.5) -> (In Range?=w801:bool)  [unwired: 1 out]
              n398 = In Range and Coerce(upper limit=22.9, x=w785, lower limit=14.5) -> (In Range?=w795:bool)  [unwired: 1 out]
              n399 = In Range and Coerce(upper limit=31.4, x=w785, lower limit=23.0) -> (In Range?=w798:bool)  [unwired: 1 out]
              n400 = In Range and Coerce(upper limit=14.4, x=w785, lower limit=1.0) -> (In Range?=w792:bool)  [unwired: 1 out]
              n401 = Concatenate Strings(w890, w789, w889, w789, w788, "\r", "\n") -> (w834:string)
              "Socket String" <- w834
              n402 = case shown="True" w873 {
                tunnel: [w965 w969] -> w875
                tunnel: w872 -> [w967 w970]
                tunnel: w834 -> [w966 w968]
                frame False {
                  # "L'array si riempie\nperchè non si è riempito di 15 elementi"
                  n403 = Build Array (concatenate)(w967, w966) -> (w965:string[])
                }
                frame True {
                  # "Ruota l'array cancellando il più vecchio dato\ne ne inserisce uno nuovo."
                  n404 = Rotate 1D Array(1:w970, 2:-1 ("n")) -> (0:w973:string[])
                  n405 = Array Size(array=w973) -> (size(s)=w972:i32)
                  n406 = Decrement(x=w972) -> (x-1=w971:i32)
                  n407 = Replace Array Subset(array=w973, new element=w968, index=w971) -> (w969:string[])
                }
              }
              "Array via socket" <- w875
              n408 = case shown="True" w801 {
                frame False {
                  w909 = u32 4914944
                  n409 = local write "37 2"(FALSE ("37")) -> ()
                  n410 = property on="37_R" class="Knob (strict)"("BGColor"=w909, "FGColor"=w909) -> ()  [unwired: 2 in, 2 out]
                }
                frame True {
                  w911 = u32 16771057
                  n411 = local write "37 2"(TRUE ("37")) -> ()
                  n412 = property on="37_R" class="Knob (strict)"("BGColor"=w911, "FGColor"=w911) -> ()  [unwired: 2 in, 2 out]
                }
              }
              n413 = case shown="True" w798 {
                frame False {
                  w905 = u32 4914944
                  n414 = local write "24 2"(FALSE ("24")) -> ()
                  n415 = property on="24_R" class="Knob (strict)"("BGColor"=w905, "FGColor"=w905) -> ()  [unwired: 2 in, 2 out]
                }
                frame True {
                  w907 = u32 16746637
                  n416 = local write "24 2"(TRUE ("24 2")) -> ()
                  n417 = property on="24_R" class="Knob (strict)"("BGColor"=w907, "FGColor"=w907) -> ()  [unwired: 2 in, 2 out]
                }
              }
              n418 = case shown="True" w795 {
                frame False {
                  w901 = u32 4914944
                  n419 = local write "12 2"(FALSE ("12")) -> ()
                  n420 = property on="12_R" class="Knob (strict)"("BGColor"=w901, "FGColor"=w901) -> ()  [unwired: 2 in, 2 out]
                }
                frame True {
                  w903 = u32 16716308
                  n421 = local write "12 2"(TRUE ("12 2")) -> ()
                  n422 = property on="12_R" class="Knob (strict)"("BGColor"=w903, "FGColor"=w903) -> ()  [unwired: 2 in, 2 out]
                }
              }
              n423 = Initialize Array(w787) -> (w869:dbl[])  [unwired: 1 in]
              n424 = case shown="True" w792 {
                frame False {
                  w897 = u32 4914944
                  n425 = local write "6 2"(FALSE ("6")) -> ()
                  n426 = property on="6_R" class="Knob (strict)"("BGColor"=w897, "FGColor"=w897) -> ()  [unwired: 2 in, 2 out]
                }
                frame True {
                  w899 = u32 13107215
                  n427 = local write "6 2"(TRUE ("6 2")) -> ()
                  n428 = property on="6_R" class="Knob (strict)"("BGColor"=w899, "FGColor"=w899, "BG Color"=w899) -> ()  [unwired: 2 in, 2 out]
                }
              }
              n429 = Decimate 1D Array(w869) -> ()  [unwired: 2 out]
              n430 = Set File Position(refnum=w870, from (0:start)=enum16{"start", "end", "current"}."current" ("pos mode (0:2)"), error in=w893) -> (refnum out=w808:refnum<file>, error out=w807:errorcluster)  [unwired: 1 in]
              n431 = Write to Binary File ("Write File")(file (use dialog)=w808, data=w834, error in=w807, 5:FALSE ("prepend array or string size? (T)")) -> (refnum out=w868:refnum<file>, error out=w866:errorcluster)  [unwired: 2 in, 1 out]
              n432 = Get Date/Time In Seconds() -> (seconds since 1Jan1904=w809:timestamp)
              n433 = case shown="True" "temp.csv midnight" {
                tunnel: w868 -> [w952 w959]
                tunnel: [w952 w964] -> w867
                tunnel: w866 -> [w951 w961]
                tunnel: [w951 w963] -> w865
                frame False {
                }
                frame True {
                  w957 = enum16{"start", "end", "current"}."start" ("pos mode (0:2)")
                  n434 = Wait (ms)(milliseconds to wait=u32 3000) -> ()  [unwired: 1 out]
                  n435 = call <vilib>:"compatCalcOffset.vi"("error in"=w961, "pos mode (0:1)"=w957, "refnum"=w959) -> ("error out"=w955:errorcluster, "offset"=w954:i32, "dup refnum"=w953:refnum<file>)  [unwired: 6 in]
                  n436 = Set File Size(4:w955, 6:w954, 7:w953) -> (0:w960:errorcluster, 3:w958:refnum<file>)
                  n437 = Set File Position(refnum=w958, from (0:start)=w957, error in=w960) -> (refnum out=w964:refnum<file>, error out=w963:errorcluster)  [unwired: 1 in]
                  n438 = property on="temp.csv midnight" class="Bool (strict)"("Value"=FALSE) -> ()  [unwired: 2 in, 2 out]
                }
              }
              n439 = call <vilib>:"LV70TimeStampToDateRec.vi"("time stamp"=w809) -> ("date time rec"=w858:T6)
              n440 = Unbundle By Name(w858) -> ("second"=w851:i32, "minute"=w852:i32, "hour"=w857:i32)
              n441 = Multiply(x=w857, y=w854) -> (x*y=w856:i32)
              n442 = Add(x=w852, y=w856) -> (x+y=w855:i32)
              n443 = Multiply(x=w855, y=w854) -> (x*y=w853:i32)
              n444 = Add(x=w851, y=w853) -> (x+y=w850:i32)
              n445 = Subtract(x=w850, y=w854) -> (x-y=w859:i32)
              n446 = Add(x=sgl 0.0, y=w859) -> (x+y=w838:sgl)
              n447 = Subtract(x=w838, y="Time Knob") -> (x-y=w849:sgl)
              n448 = Refnum to Path(1:w863) -> (0:w835:path)
              n449 = Build Array(w838, w787) -> (w862:dbl[])
              n450 = case shown="True" "Graph" {
                tunnel: w849 -> [_ w929]
                tunnel: w838 -> [_ w937]
                tunnel: "Time Knob" -> [_ w932]
                frame False {
                }
                frame True {
                  # "Impostazioni grafico principale"
                  # "Scala dei kV/m sul grafico"
                  n451 = control-ref of="FEM Graph"() -> (w938:refnum<vi>)
                  n452 = Multiply(x="kV/m knob", y=-1) -> (x*y=w940:sgl)
                  n453 = property on="Property Node" class="XYGraph (strict)"(reference=w938, "Y Scale.Range:Minimum"=w940, "Y Scale.Range:Maximum"="kV/m knob") -> ()  [unwired: 1 in, 2 out]
                  n454 = Equal?(x=w932, y=86400) -> (x = y?=w931:bool)
                  n455 = case shown="True" w931 {
                    tunnel: [w941 300] -> w930
                    tunnel: w929 -> [w941 _]
                    frame False {
                    }
                    frame True {
                    }
                  }
                  n456 = property on="Property Node" class="XYGraph (strict)"(reference=w938, "X Scale.Range:Minimum"=w930, "X Scale.Range:Maximum"=w937, "X Scale.Range:Increment"=w937, "X Scale.Style"=u8 6, "X Scale.Uniform Marker Spacing?"=TRUE) -> ()  [unwired: 1 in, 2 out]
                }
              }
              n457 = Get Date/Time In Seconds() -> (seconds since 1Jan1904=w848:timestamp)
              n458 = File/Directory Info(path=w835) -> (last mod=w847:timestamp)  [unwired: 1 in, 6 out]
              n459 = Subtract(x=w848, y=w847) -> (x-y=w846:dbl)
              n460 = Less?(x=w846, y=86400.0) -> (x < y?=w844:bool)
              n461 = case shown="True" w844 {
                tunnel: [FALSE ("append to file? (new file:F)") TRUE ("append to file? (new file:F)")] -> w861
                frame False {
                }
                frame True {
                }
              }
              n462 = call-poly <vilib>:"Write To Spreadsheet File.vi"("append to file? (new file:F)"=w861, "1D data"=w862, "file path (dialog if empty)"=w835) -> ("new file path (Not A Path if cancelled)"=w820:path)  [unwired: 5 in]
              n463 = File/Directory Info(path=w820) -> (size=w810:i64)  [unwired: 1 in, 6 out]
              n464 = To Long Integer(number=w810) -> (32bit integer=w813:i32)
              n465 = Subtract(x=w813, y=6010) -> (x-y=w828:i32)
              n466 = Subtract(x=w813, y=36000) -> (x-y=w823:i32)
              n467 = call-poly <vilib>:"Read From Spreadsheet File.vi"("start of read offset (chars.:0)"=w828, "file path (dialog if empty)"=w820) -> ("all rows"=w812:dbl[][])  [unwired: 5 in, 4 out]
              n468 = call-poly <vilib>:"Read From Spreadsheet File.vi"("start of read offset (chars.:0)"=w823, "file path (dialog if empty)"=w820) -> ("all rows"=w822:dbl[][])  [unwired: 5 in, 4 out]
              n469 = for {
                tunnel: w812 -> [w925] mode=indexing
                tunnel: [w924] -> w827 mode=indexing
                # "Lettura del file graph.txt\nper media 10 min"
                n470 = Index Array(array=w925, index=1) -> (element=w924:dbl)
              }
              n471 = for {
                tunnel: w822 -> [w922] mode=indexing
                tunnel: [w921] -> w821 mode=indexing
                # "Lettura del file graph.txt\nper media 1 ora"
                n472 = Index Array(array=w922, index=1) -> (element=w921:dbl)
              }
              n473 = call-poly <vilib>:"Read From Spreadsheet File.vi"("file path (dialog if empty)"=w820) -> ("all rows"=w833:dbl[][])  [unwired: 6 in, 4 out]
              n474 = for {
                tunnel: w833 -> [w946] mode=indexing
                tunnel: [w948] -> w837 mode=indexing
                tunnel: [w945] -> w830 mode=indexing
                # "Lettura del file graph.txt\ne rimpimento grafici"
                n475 = Index Array(array=w946, index #1=0 ("index"), index #2=1 ("index")) -> (element #1=w947:dbl, element #2=w945:dbl)
                n476 = Bundle(w947, w945) -> (w948:cluster{dbl, dbl})  [unwired: 1 in]
              }
              "FEM Graph_IMAGES" <- w837
              "FEM Graph" <- w837
              n477 = Array Max & Min(array=w830) -> (max value=→"Max":dbl, min value=→"Min":dbl)  [unwired: 2 out]
              n478 = Array Max & Min(array=w827) -> (max value=→"Max":dbl, min value=→"Min":dbl)  [unwired: 2 out]
              n479 = Array Max & Min(array=w821) -> (max value=→"Max":dbl, min value=→"Min":dbl)  [unwired: 2 out]
              n480 = Less Or Equal?(x=w838, y=4) -> (x <= y?=w840:bool)
              n481 = Greater Or Equal?(x=w838, y=1) -> (x >= y?=w839:bool)
              n482 = And(x=w840, y=w839) -> (x .and. y?=w836:bool)
              n483 = case shown="True" w836 {
                tunnel: w835 -> [_ w927]
                frame False {
                  n484 = property on="FEM Graph" class="XYGraph (strict)" props=["Visible"]() -> ()  [unwired: 2 in, 3 out]
                }
                frame True {
                  n485 = call <vilib>:"compatOverwrite.vi"("overwrite (F)"=TRUE) -> ("overwrite?"=w926:T1)
                  n486 = Open/Create/Replace File(file path (use dialog)=w927, operation (0:open)=w926) -> ()  [unwired: 4 in, 3 out]
                }
              }
            }
            n487 = node-c288(w390) -> ()  [unwired: 1 out]
            n488 = node-c288(30000) -> (w386:T2)  [unwired: 3 in]
            n489 = while {
              stop <- TRUE continue-if-true
              # "Led acceso per 60 sec"
              # "Alert distanza\nfulmini"
              n490 = case shown="True" "37 2" {
                frame False {
                }
                frame True {
                  n491 = Wait (ms)(milliseconds to wait=u32 60000) -> ()  [unwired: 1 out]
                }
              }
              n492 = Wait Until Next ms Multiple(millisecond multiple=250) -> ()  [unwired: 1 out]
              "37" <- "37 2"
            }
            n493 = timed-loop {
              timing: w386 -> [_]
              timing-out: [_] -> w385
              tunnel: w383 -> [w421]
              stop <- _ continue-if-true
              # "Creazionee fieldmill_tmp.png"
              n494 = node-c288() -> ()  [unwired: 1 in, 1 out]
              n495 = Current VI's Path() -> (path=w427:path)
              n496 = Open VI Reference(vi path=w427) -> (vi reference=w426:refnum<vi>)  [unwired: 5 in, 1 out]
              n497 = invoke class="VI" method="FP.Get Image"(reference=w426) -> (reference out=w425:refnum<vi>, "image data"=w424:T7)  [unwired: 5 in, 4 out]
              n498 = Strip Path(path=w421) -> (stripped path=w423:path)  [unwired: 1 out]
              n499 = Build Path(base path=w423, name or relative path="efieldmill_tmp.png") -> (appended path=w420:path)
              n500 = Close Reference(reference=w425) -> ()  [unwired: 1 in, 1 out]
              n501 = call <vilib>:"Write PNG File.vi"("image data"=w424, "path to PNG file"=w420) -> ()  [unwired: 8 in, 2 out]
              n502 = node-c288() -> ()  [unwired: 1 in, 1 out]
            }
            n503 = while {
              stop <- TRUE continue-if-true
              w637 = "\n"
              w638 = "\r"
              # "Stringa da inviare via socket.\n15 stringhe con LF in mezzo."
              n504 = local read "Array via socket"() -> (w634:string[])
              n505 = Array To Cluster(array=w634) -> (cluster=w633:T8)
              n506 = Unbundle(w633) -> ("Array via socket[0]"=w668:string, "Array via socket[1]"=w667:string, "Array via socket[2]"=w651:string, "Array via socket[3]"=w650:string, "Array via socket[4]"=w649:string, "Array via socket[5]"=w648:string, "Array via socket[6]"=w647:string, "Array via socket[7]"=w646:string, "Array via socket[8]"=w645:string, "Array via socket[9]"=w644:string, "Array via socket[10]"=w643:string, "Array via socket[11]"=w642:string, "Array via socket[12]"=w641:string, "Array via socket[13]"=w640:string, "Array via socket[14]"=w639:string)
              n507 = Search/Split String(string=w668, search string/char (-)=w638) -> (substring before match=w666:string)  [unwired: 1 in, 2 out]
              n508 = Search/Split String(string=w667, search string/char (-)=w638) -> (substring before match=w665:string)  [unwired: 1 in, 2 out]
              n509 = Search/Split String(string=w651, search string/char (-)=w638) -> (substring before match=w664:string)  [unwired: 1 in, 2 out]
              n510 = Search/Split String(string=w650, search string/char (-)=w638) -> (substring before match=w663:string)  [unwired: 1 in, 2 out]
              n511 = Search/Split String(string=w649, search string/char (-)=w638) -> (substring before match=w662:string)  [unwired: 1 in, 2 out]
              n512 = Search/Split String(string=w648, search string/char (-)=w638) -> (substring before match=w661:string)  [unwired: 1 in, 2 out]
              n513 = Search/Split String(string=w647, search string/char (-)=w638) -> (substring before match=w660:string)  [unwired: 1 in, 2 out]
              n514 = Search/Split String(string=w646, search string/char (-)=w638) -> (substring before match=w659:string)  [unwired: 1 in, 2 out]
              n515 = Search/Split String(string=w645, search string/char (-)=w638) -> (substring before match=w658:string)  [unwired: 1 in, 2 out]
              n516 = Search/Split String(string=w644, search string/char (-)=w638) -> (substring before match=w657:string)  [unwired: 1 in, 2 out]
              n517 = Search/Split String(string=w643, search string/char (-)=w638) -> (substring before match=w656:string)  [unwired: 1 in, 2 out]
              n518 = Search/Split String(string=w642, search string/char (-)=w638) -> (substring before match=w655:string)  [unwired: 1 in, 2 out]
              n519 = Search/Split String(string=w641, search string/char (-)=w638) -> (substring before match=w654:string)  [unwired: 1 in, 2 out]
              n520 = Search/Split String(string=w640, search string/char (-)=w638) -> (substring before match=w653:string)  [unwired: 1 in, 2 out]
              n521 = Search/Split String(string=w639, search string/char (-)=w638) -> (substring before match=w652:string)  [unwired: 1 in, 2 out]
              n522 = Wait Until Next ms Multiple(millisecond multiple=250) -> ()  [unwired: 1 out]
              n523 = Concatenate Strings(w666, w637, w665, w637, w664, w637, w663, w637, w662, w637, w661, w637, w660, w637, w659, w637, w658, w637, w657, w637, w656, w637, w655, w637, w654, w637, w653, w637, w652, w637) -> (→"Multi socket String":string)
            }
            n524 = while {
              stop <- TRUE continue-if-true
              # "Led acceso per 60 sec"
              # "Alert distanza\nfulmini"
              n525 = case shown="True" "24 2" {
                frame False {
                }
                frame True {
                  n526 = Wait (ms)(milliseconds to wait=u32 60000) -> ()  [unwired: 1 out]
                }
              }
              n527 = Wait Until Next ms Multiple(millisecond multiple=250) -> ()  [unwired: 1 out]
              "24" <- "24 2"
            }
            n528 = while {
              stop <- TRUE continue-if-true
              # "Led acceso per 60 sec"
              # "Alert distanza\nfulmini"
              n529 = case shown="True" "12 2" {
                frame False {
                }
                frame True {
                  n530 = Wait (ms)(milliseconds to wait=u32 60000) -> ()  [unwired: 1 out]
                }
              }
              n531 = Wait Until Next ms Multiple(millisecond multiple=250) -> ()  [unwired: 1 out]
              "12" <- "12 2"
            }
            n532 = node-c288(w385) -> ()  [unwired: 1 out]
            n533 = while {
              stop <- TRUE continue-if-true
              # "Led acceso per 60 sec"
              # "Alert distanza\nfulmini"
              n534 = case shown="True" "6 2" {
                frame False {
                }
                frame True {
                  n535 = Wait (ms)(milliseconds to wait=u32 60000) -> ()  [unwired: 1 out]
                }
              }
              n536 = Wait Until Next ms Multiple(millisecond multiple=250) -> ()  [unwired: 1 out]
              "6" <- "6 2"
            }
          }
        }
        n537 = case shown="No Error" w349 {
          tunnel: w349 -> [w355 _]
          tunnel: w353 -> [_ w360]
          tunnel: w352 -> [_ w359]
          tunnel: w345 -> [_ w358]
          frame Error {
            w357 = T5 0 items=["no dialog", "OK message", "continue or stop message", "OK message + warnings", "continue/stop + warnings"] ("type of dialog (OK msg:1)")
            n538 = call <vilib>:"Simple Error Handler.vi"("type of dialog (OK msg:1)"=w357, "error in (no error)"=w355) -> ("message"=w356:string)  [unwired: 3 in, 4 out]
            n539 = local write "COM err msg: 2"(w356) -> ()
          }
          frame No Error {
            n540 = while {
              tunnel: w360 -> [w368]
              tunnel: w359 -> [w363]
              tunnel: w358 -> [w364]
              stop <- TRUE continue-if-true
              w370 = T5 0 items=["no dialog", "OK message", "continue or stop message", "OK message + warnings", "continue/stop + warnings"] ("type of dialog (OK msg:1)")
              w373 = u32 500  # Output Rate
              # "Più ripetizioni"
              n541 = property on="Mediated v." class="Bool (strict)"() -> ("Value"=w362:bool)  [unwired: 2 in, 2 out]
              n542 = case shown="False" w362 {
                tunnel: [w374 w376] -> w365
                tunnel: w364 -> [w375 _]
                tunnel: w363 -> [_ w377]
                frame True {
                  # "Coda kV/m mediati"
                  n543 = Dequeue Element(queue=w375) -> (element=w374:string)  [unwired: 2 in, 3 out]
                  "kV/m" <- w374
                }
                frame False {
                  # "Coda kV/m"
                  n544 = Dequeue Element(queue=w377) -> (element=w376:string)  [unwired: 2 in, 3 out]
                  n545 = local write "kV/m"(w376) -> ()
                }
              }
              n546 = call "BoltekStr.vi"("Arrivo Kv/m"=w365) -> ("String Boltek"=w366:string)
              n547 = Concatenate Strings(w366, w366, w366, w366, w366, w366, w366, w366, w366, w366) -> (w367:string)
              "data string 3" <- w367
              n548 = VISA Write(VISA resource name=w368, write buffer=w367) -> (error out=w369:errorcluster)  [unwired: 1 in, 2 out]
              n549 = Wait (ms)(milliseconds to wait=w373) -> ()  [unwired: 1 out]
              n550 = Unbundle By Name(w369) -> ("code"=w372:i32)
              n551 = call <vilib>:"Simple Error Handler.vi"("error code (no error:0)"=w372, "type of dialog (OK msg:1)"=w370) -> ("message"=→"COM err msg: 2":string)  [unwired: 3 in, 4 out]
            }
          }
        }
      }
      frame #4 {
        n552 = VISA Close(VISA resource name=w1054) -> ()  [unwired: 1 in, 1 out]
        n553 = VISA Close(VISA resource name=w1055) -> ()  [unwired: 1 in, 1 out]
      }
    }
  }
  n554 = VISA Unlock(11:w107) -> (3:w108:refnum<visa-resource-name>)  [unwired: 1 in, 1 out]
  n555 = VISA Close(VISA resource name=w108) -> ()  [unwired: 1 in, 1 out]
  n556 = Close File(refnum=w141, error in=w142) -> (error out=w190:errorcluster)  [unwired: 1 out]
  n557 = VISA Unlock(11:w109) -> (3:w110:refnum<visa-resource-name>)  [unwired: 1 in, 1 out]
  n558 = VISA Close(VISA resource name=w110) -> ()  [unwired: 1 in, 1 out]
  n559 = call <vilib>:"Simple Error Handler.vi"("error in (no error)"=w190) -> ()  [unwired: 4 in, 5 out]
  n560 = call "LoadSetup.vi"("section"=w32, "key"="OFFSET", "error in (not an error)"=w26) -> ("error out"=w31:errorcluster, "value"=w24:string)  [unwired: 2 in]
  n561 = Decimal String To Number(string=w24) -> (number=w23:i32)  [unwired: 2 in, 1 out]
  "Offset_p" <- w23
  n562 = Not Equal To 0?(x=w23) -> (x != 0?=w22:bool)
  n563 = call "LoadSetup.vi"("section"=w32, "key"="INVERTED", "error in (not an error)"=w31) -> ("error out"=w30:errorcluster, "value"=w20:string)  [unwired: 2 in]
  "Inverted_p" <- w20
  n564 = Not Equal?(x=w20, y="") -> (x != y?=w21:bool)
  n565 = And(x=w22, y=w21) -> (x .and. y?=w18:bool)
  n566 = call "LoadSetup.vi"("section"=w32, "key"="MEDIATED", "error in (not an error)"=w30) -> ("error out"=→"Errori lettura file di configurazione":errorcluster, "value"=w15:string)  [unwired: 2 in]
  "Mediated_p" <- w15
  n567 = Not Equal?(x=w15, y="") -> (x != y?=w16:bool)
  n568 = And(x=w18, y=w16) -> (x .and. y?=w14:bool)
  n569 = case shown="False" w14 {
    frame False {
      n570 = property on="MENU FILTERS" class="Bool"("Disabled"=u8 0) -> ()  [unwired: 2 in, 2 out]
    }
    frame True {
      n571 = property on="MENU FILTERS" class="Bool"("Disabled"=u8 2) -> ()  [unwired: 2 in, 2 out]
    }
  }
